vi "SQL_SearchSpareParts.vi"() -> (1 "`Location.Text":string, 2 "Description.Text":string, 3 "ToolCribPN.Text":string)   [LabVIEW 2017]
panel:
  out "ResultQueryString":string
  in  "stop":bool
  in  "Selector":u16(ring)=1 items=["Model", "Make", "ToolCribPN", "Description"]
  in  "Location":u16(ring) items=["12-A-10", "11-B-02", "16-A-03", "15-A-09", "ZARA-A-04", "13-C-02", "11-D-04", "ZARA-A-02", "11-A-02", "RACK-D-06", "11-B-02", "16-A-03", "ZARA-C-08", "ZARA-B-11", "ZARA-B-11", "11-D-09", "15-A-09", "15-A-09", "11-C-04", "ZARA-C-02", "18-C-02", "18-C-02", "18-C-02", "18-C-03", "18-C-03", "18-C-03", "18-C-02", "18-C-05", "ZARA-C-05", "ZARA-C-04", "18-C-03", "18-C-03", "18-C-03", "18-C-03", "18-C-03", "18-C-07", "18-C-07", "15-A-03", "15-C-08", "ZARA-C-09", "ZARA-B-02", "ZARA-B-03", "18-C-14", "RACK-30B-6", "18-C-12", "18-C-14", "18-C-13", "ZARA-B-02", "CARRO-J-02", "ZARA-C-04", "15-C-07", "18-C-14", "18-C-07", "18-C-07", "RACK-30A-1", "11-B-05", "GAV,PAPELE", "16-A-04", "11-B-05", "11-B-06", "11-B-06", "RACK30F-08", "ZARA-A-10", "15-C-11", "15-C-05", "15-B-08", "RACK30C-07", "18-C-07", "15-C-11", "11-C-07", "16-A-12", "16-A-05", "16-A-01", "RACK-7-04", "16-A-09", "15-B-6", "CARRO-B-06", "11-B-03", "ZARA-B-10", "11-B-03", "15-A-16", "15-B-03", "11-B-02", "16-A-01", "15-B-11", "16-A-09", "15-B-11", "15-B-11", "15-B-11", "15-B-12", "15-B-12", "15-A-17", "RACK-30G-4", "11-C-05", "15-B-11", "15-B-11", "RACK-30A-7", "15-B-12", "16-A-04", "RACK-30G-4", "18-C-03", "15-B-03", "11-C-05", "19-D-05", "18-C-07", "16-A-07", "19-A-05", "18-M-05", "19-A-01", "19-A-01", "19-A-01", "19-A-01", "19-A-01", "19-A-01", "19-A-01", "16-A-01", "15-A-01", "19-A-08", "19-A-01", "19-A-01", "19-A-01", "19-A-01", "19-A-01", "19-A-01", "19-A-01", "19-A-01", "19-A-01", "18-C-14", "19-A-02", "19-A-07", "11-D-03", "15-C-03", "18-C-13", "19-A-07", "18-C-14", "19-A-03", "19-A-02", "15-A-01", "16-A-01", "19-D-01", "19-A-02", "19-A-02", "19-A-02", "19-A-03", "19-A-02", "19-A-02", "15-B-10", "15-B-10", "15-B-10", "19-D-07", "19-D-07", "11-D-01", "19-C-01", "19-C-01", "19-C-01", "19-C-01", "19-C-01", "19-C-01", "19-D-03", "19-D-03", "19-D-03", "19-D-03", "19-D-03", "19-D-03", "19-D-03", "16-A-01", "19-D-03", "19-D-03", "19-D-03", "19-D-03", "19-D-03", "19-D-03", "19-D-03", "19-D-03", "19-D-03", "19-D-03", "19-D-03", "19-D-03", "19-D-03", "19-D-03", "19-D-03", "19-D-03", "19-D-08", "19-D-02", "19-D-06", "19-D-05", "19-D-06", "ZARA-L-18", "19-A-03", "19-A-03", "19-D-03", "19-D-03", "19-A-03", "19-A-03", "15-B-08", "19-A-11", "19-A-03", "19-A-03", "19-A-03", "19-A-03", "19-A-06", "RACK-5E-02", "19-B-04", "19-B-07", "PENT.", "18-C-05", "PENT.", "19-A-03", "19-A-03", "15-B-07", "18-M-02", "19-A-03", "19-A-03", "19-A-03", "19-D-10", "19-A-02", "19-A-05", "19-A-05", "19-D-09", "19-A-07", "15-A-04", "15-A-04", "19-D-04", "RACK33B-03", "ZARA-K-12", "15-C-01", "ZARA-K-17", "15-C-01", "15-C-01", "19-A-03", "19-A-04", "19-A-04", "15-B-11", "19-A-04", "19-A-04", "19-A-04", "19-A-10", "19-A-04", "19-D-02", "CARRO-B-03", "15-B-05", "11-C-01", "ZARA-K-08", "ZARA-K-08", "ZARA-K-08", "11-C-01", "ZARA-K-08", "11-C-01", "ZARA-K-12", "11-C-01", "15-C-01", "ZARA-K-18", "ZARA-K-16", "ZARA-K-08", "19-A-05", "11-C-01", "15-B-04", "19-C-02", "15-C-05", "17-D-11", "GAV QUIM 1", "15-B-10", "17-D-08", "17-D-11", "15-C-04", "15-B-01", "15-B-04", "11-G-01", "11-G-01", "11-G-01", "18-C-14", "ZARA-S-03", "15-C-02", "17-D-01", "15-A-02", "19-A-04", "19-A-04", "18-C-05", "19-A-04", "18-C-05", "18-C-05", "18-M-03", "RACK-4D-01", "RACK30G-03", "19-A-04", "19-A-04", "19-A-04", "CARRO-H-03", "RACK-11K-8", "CARRO-B-01", "15-B-06", "19-A-11", "19-A-09", "18-M-01", "19-A-11", "15-B-11", "ZARA-K-22", "CARRO-H-02", "ZARA-L-05", "RACK33B-02", "RACK33B-02", "RACK33B-02", "CARRO-A-06", "CARRO-A-06", "CARTO-QUIM", "ZARA-K-09", "ZARA-L-05", "ZARA-L-05", "ZARA-L-05", "CARRO-A-03", "19-A-02", "CARRO-A-06", "CARRO-A-06", "CARRO-A-06", "ZARA-V-02", "ZARA-V-02", "ZARA-K-20", "ZARA-E-02", "CARRO-L-03", "ZARA-K-16", "ZARA-K-07", "19-C-06", "CARRO-A-06", "19-C-06", "CARRO-A-06", "CARRO-A-06", "ZARA-K-21", "ZARA-K-20", "19-B-04", "CARRO-H-03", "RACK-33A-1", "ZARA-K-16", "ZARA-K-16", "19-C-04", "19-C-04", "CARRO-H-02", "ZARA-L-05", "18-M-01", "11-B-08", "16-A-02", "CARRO-H-04", "ZARA-T-01", "ZARA-S-05", "ZARA-S-05", "ZARA-U-03", "ZARA-K-06", "ZARA-K-05", "13-C-02", "ZARA-L-16", "ZARA-D-01", "18-M-02", "CARRO-B-05", "15-A-07", "11-C-07", "CARRO-A-12", "15-C-02", "ZARA-L-17", "CARRO-B-12", "ZARA-T-02", "ZARA-L-05", "ZARA-Q-03", "ZARA-F-02", "ZARA-F-02", "ZARA-K-20", "11-D-01", "ZARA-K-14", "11-D-02", "ZARA-K-13", "ZARA-K-06", "ZARA-L-17", "ZARA-K-06", "ZARA-K-06", "ZARA-K-13", "ZARA-K-06", "ZARA-K-16", "ZARA-K-16", "ZARA-K-18", "ZARA-K-05", "ZARA-D-02", "ZARA-K-05", "ZARA-K-05", "CARRO-A-05", "ZARA-K-05", "ZARA-K-05", "11-B-03", "ZARA-K-18", "ZARA-L-02", "CARRO-I-01", "ZARA-L-16", "ZARA-L-02", "ZARA-K-13", "11-D-02", "15-B-04", "13-C-03", "ZARA-V-02", "ZARA-U-09", "17-D-02", "CARRO-H-04", "ZARA-L-01", "ZARA-K-08", "15-B-10", "ZARA-D-03", "ZARA-L-01", "ZARA-K-12", "15-A-04", "15-B-07", "ZARA-D-02", "11-G-01", "CARRO-G-03", "11-D-02", "CARRO-G-03", "ZARA-K-06", "ZARA-J-02", "ZARA-K-06", "ZARA-K-11", "ZARA-S-03", "11-D-02", "ZARA-K-13", "ZARA-U-06", "ZARA-K-13", "ZARA-K-13", "15-B-06", "ZARA-L-13", "11-B-02", "11-B-02", "11-C-07", "11-C-07", "11-D-01", "11-C-07", "11-D-01", "11-D-01", "ZARA-L-04", "ZARA-K-10", "ZARA-L-13", "11-C-01", "11-D-02", "ZARA-L-04", "ZARA-L-07", "ZARA-K-14", "11-D-01", "15-B-05", "ZARA-K-10", "ZARA-M-04", "15-C-02", "ZARA-K-14", "ZARA-M-04", "ZARA-M-04", "ZARA-M-04", "ZARA-M-04", "ZARA-M-04", "ZARA-K-21", "15-C-02", "ZARA-D-06", "ZARA-L-06", "ZARA-L-06", "ZARA-L-06", "15-B-06", "15-B-05", "15-B-05", "CARRO-G-05", "18-C-06", "ZARA-J-05", "19-D-01", "ZARA-Q-04", "18-C-09", "CARRO-A-01", "11-C-01", "CARRO-J-02", "CARRO-H-03", "CARRO-L-03", "CARRO-H-03", "CARRO-L-03", "ZARA-P-06", "ZARA-K-10", "ZARA-L-08", "CARRO-E-02", "ZARA-L-03", "ZARA-Q-04", "11-C-01", "ZARA-M-08", "CARRO-G-10", "CARRO-G-10", "CARRO-G-10", "CARRO-G-10", "11-A-06", "ZARA-S-03", "ZARA-U-09", "ZARA-L-13", "ZARA-L-10", "ZARA-K-06", "CARRO-B-02", "CARRO-H-03", "ZARA-L-01", "ZARA-K-14", "CARRO-G-10", "ZARA-M-08", "PENT.", "ZARA-F05-1", "17-D-01", "14-B-06", "ZARA-K-22", "ZARA-L-15", "G.QUIMICOS", "18-M-04", "RACK30F-06", "15-C-06", "15-A-17", "11-G-04", "ZARA-K-17", "ZARA-K-11", "18-M-01", "RACK30C-04", "11-B-06", "17-D-06", "RACK30F-06", "GAV1,QUIMI", "18-M-03", "15-C-11", "11-B-04", "15-A-02", "15-A-04", "RACK-3C-02", "ZARA-L-15", "RACK-4D-07", "17-D-05", "15-C-04", "15-A-01", "RACK-D4-07", "18-C-10", "CARRO-B-10", "CARRO-B-10", "CARRO-B-10", "CARRO-B-10", "ZARA-L-05", "CARRO-B-10", "RACK-D4-03", "ZARA-L-10", "11-C-03", "18-M-04", "18-C-10", "15-C-04", "CARRO-G-01", "17-D-11", "11-C-01", "11-C-03", "15-C-10", "15-A-01", "ZARA-K-16", "14-B-05", "17-D-06", "ZARA-L-16", "11-B-04", "17-D-10", "15-B-10", "ZARA-C-01", "RACK-5E-01", "15-A-14", "ZARA-L-10", "ZARA-L-10", "ZARA-L-10", "ZARA-Q-04", "15-C-03", "15-C-03", "11-C-06", "ZARA-L-15", "13-C-05", "ZARA-L-14", "ZARA-M-05", "ZARA-F-16", "17-D-02", "15-A-08", "17-D-01", "17-D-01", "ZARA-L-10", "17-D-01", "RACK-B-00", "RACK-B-00", "RACK-B-00", "11-C-01", "CARRO-A-04", "17-D-06", "15-B-08", "15-B-08", "15-B-08", "15-B-08", "19-D-04", "19-D-04", "17-D-08", "13-C-01", "13-C-01", "ZARA-L-07", "15-B-03", "11-B-04", "18-C-06", "17-D-01", "ZARA-L-15", "ZARA-L-15", "11-B-04", "15-A-11", "ZARA-M-08", "ZARA-K-15", "14-B-09", "17-D-02", "18-M-03", "15-B-02", "15-B-02", "15-B-02", "ZARA-M-06", "ZARA-S-04", "17-D-02", "ZARA-L-19", "GAV-QUIM1", "15-C-06", "18-C-06", "CARRO-C-02", "CARRO-C-02", "ZARA-J-01", "11-B-08", "ZARA-M-03", "ZARA-F-17", "ZARA-M-03", "ZARA-M-03", "ZARA-J-01", "ZARA-E-04", "ZARA-M-10", "ZARA-M-08", "ZARA-M-08", "15-B-02", "15-B-02", "15-B-02", "ZARA-J-01", "12-A-10", "15-B-11", "15-C-05", "11-A-02", "14-B-09", "CARRO-G-06", "CARRO-G-06", "15-C-07", "14-B-09", "11-A-02", "CARRO-G-06", "11-A-02", "CARRO-G-06", "ZARA-J-01", "ZARA-M-10", "CARRO-A-04", "CARRO-G-06", "CARRO-A-04", "ZARA-P-04", "CARRO-G-06", "11-D-04", "11-D-04", "11-D-04", "CARRO-A-04", "CARRO-A-04", "CARRO-G-06", "11-B-07", "PENDIENTE", "PENDIENTE", "CARRO-C-04", "ZARA-M-10", "14-B-05", "CARRO-A-02", "CARRO-A-02", "14-B-09", "CARRO-B-12", "CARRO-J-02", "15-C-06", "15-C-04", "ZARA-K-07", "CUARTO NUV", "ZARA-P-05", "ZARA-N-13", "ZARA-N-03", "ZARA-N-04", "ZARA-N-02", "ZARA-O-11", "ZARA-M-10", "CARRO-A-01", "15-B-02", "11-C-02", "ZARA-N-01", "ZARA-N-01", "ZARA-N-01", "ZARA-N-01", "ZARA-N-01", "15-A-16", "11-D-02", "RACK-D-5", "ZARA-N-12", "ZARA-N-12", "18-C-08", "18-C-08", "CARRO-B-03", "12-A-05", "15-C-04", "15-C-04", "11-D-10", "ZARA-N-01", "18-M-07", "ZARA-N-13", "ZARA-N-13", "ZARA-T-06", "ZARA-T-06", "ZARA-T-06", "ZARA-T-06", "ZARA-T-06", "ZARA-T-06", "ZARA-O-14", "CARRO-A-03", "CARRO-A-03", "CARRO-A-03", "CARRO-A-03", "CARRO-A-03", "CARRO-A-03", "CARRO-A-03", "CARRO-A-03", "CARRO-A-03", "CARRO-A-03", "CARRO-A-03", "CARRO-A-03", "CARRO-A-03", "ZARA-N-04", "ZARA-N-04", "CARRO-A-03", "CARRO-A-03", "CARRO-A-03", "11-C-01", "11-C-02", "11-C-02", "ZARA-N-12", "ZARA-N-04", "ZARA-N-04", "ZARA-N-04", "ZARA-N-12", "11-C-01", "CARRO-A-03", "ZARA-T-06", "ZARA-T-06", "ZARA-T-06", "ZARA-T-06", "ZARA-T-06", "CARRO-A-03", "11-D-01", "11-D-01", "11-C-06", "11-D-01", "CARRO-A-03", "CARRO-B-05", "15-C-03", "11-D-02", "ZARA-P-04", "ZARA-O-09", "ZARA-N-13", "ZARA-N-13", "ZARA-N-13", "ZARA-P-02", "ZARA-N-15", "ZARA-U-01", "11-B-05", "CARRO-A-04", "ZARA-P-04", "ZARA-O-13", "ZARA-O-13", "ZARA-O-14", "ZARA-O-13", "ZARA-O-13", "ZARA-O-13", "ZARA-O-13", "11-C-01", "ZARA-T-07", "ZARA-T-07", "ZARA-T-07", "ZARA-T-07", "ZARA-T-07", "ZARA-T-07", "CARRO-L-02", "CARRO-L-02", "ZARA-T-03", "ZARA-P-04", "ZARA-O-13", "CARRO-B-12", "17-D-07", "ZARA-T-07", "ZARA-T-07", "CARRO-K-06", "CARRO-K-09", "ZARA-T-03", "ZARA-T-03", "ZARA-T-06", "ZARA-T-04", "ZARA-T-04", "ZARA-T-04", "ZARA-T-04", "ZARA-T-04", "ZARA-T-04", "CARRO-B-12", "CARRO-B-12", "CARRO-B-12", "CARRO-B-12", "ZARA-T-04", "ZARA-T-04", "ZARA-T-04", "ZARA-T-05", "ZARA-T-05", "ZARA-T-05", "ZARA-T-05", "ZARA-T-05", "ZARA-T-07", "ZARA-T-07", "ZARA-T-07", "ZARA-T-07", "ZARA-T-07", "ZARA-T-07", "ZARA-T-07", "15-A-16", "13-C-03", "CARRO-B-04", "CARRO-A-02", "CARRO-A-02", "11-D-03", "ZARA-U-01", "ZARA-T-09", "CARRO-H-03", "17-D-02", "ZARA-U-04", "ZARA-U-04", "ZARA-U-04", "ZARA-U-04", "ZARA-U-04", "ZARA-U-04", "CARRO-K-02", "CARRO-K-02", "ZARA-U-04", "CARRO-K-09", "ZARA-U-04", "ZARA-U-04", "ZARA-T-02", "18-C-17", "CARRO-K-09", "11-D-03", "RACK30B-07", "11-B-03", "CARRO-K-09", "CARRO-B-11", "CARRO-B-11", "CARRO-B-11", "CARRO-B-11", "CARRO-B-11", "CARRO-G-09", "CARRO-G-09", "CARRO-G-09", "CARRO-G-09", "CARRO-C-05", "15-B-06", "CARRO-G-08", "15-A-04", "CARRO-G-12", "CARRO-B-07", "11-D-07", "14-B-02", "11-D-04", "PEND.", "15-B-08", "15-B-08", "CARRO-G-11", "11-D-02", "CARRO-G-01", "11-D-02", "CARRO-G-11", "CARRO-G-11", "CARRO-G-12", "CARRO-G-12", "PEND.", "PEND.", "15-B-07", "CARRO-G-12", "CARRO-K-05", "CARRO-K-05", "RACK33B-02", "15-B-06", "CARRO-A-10", "CARRO-A-10", "CARRO-A-11", "CARRO-A-11", "CARRO-A-11", "CARRO-A-11", "CARRO-G-07", "CARRO-G-07", "CARRO-G-07", "CARRO-G-07", "CARRO-G-07", "CARRO-G-07", "CARRO-G-07", "18-C-03", "RACK-I-04", "CARRO-B-07", "CARRO-B-07", "CARRO-A-12", "CARRO-A-12", "CARRO-A-12", "11-D-07", "15-B-08", "11-D-03", "18-M-08", "11-D-07", "18-M-09", "15-B-08", "CARRO-B-10", "CARRO-G-11", "CARRO-G-11", "CARRO-B-04", "CARRO-G-06", "CARRO-G-11", "CARRO-G-06", "ZARA-O-04", "EN CUARTO", "CARRO-D-03", "CARRO-G-11", "15-B-02", "ZARA-O-04", "19-C-02", "ZARA-P-07", "ZARA-O-04", "CARRO-B-10", "18-C-10", "CARRO-K-05", "CARRO-K-05", "CARRO-K-05", "CARRO-K-05", "CARRO-K-05", "CARRO-K-05", "CARRO-K-05", "CARRO-K-05", "CARRO-K-05", "15-C-04", "ZARA-Q-09", "PENDIENTE", "CARRO-B-06", "CARRO-B-06", "CARRO-K-03", "CARRO-K-05", "CARRO-K-05", "CARRO-K-05", "CARRO-K-05", "CARRO-K-05", "CARRO-K-05", "CARRO-K-05", "CARRO-A-08", "PEND.", "CARRO-B-09", "CARRO-K-07", "ZARA-Q-09", "CARRO-K-03", "CARRO-K-03", "15-C-04", "15-B-03", "11-B-05", "CARRO-K-05", "CARRO-K-06", "PEND.", "PEND.", "15-B-09", "CARRO-A-07", "CARRO-A-07", "CARRO-A-07", "CARRO-A-07", "CARRO-A-07", "CARRO-A-07", "CARRO-A-07", "CARRO-A-07", "ZARA-W-04", "PEND.", "ZT-***", "CARRO-K-09", "CARRO-K-09", "ZARA-E-01", "ZARA-E-01", "ZARA-E-03", "ZARA-E-01", "ZARA-E-01", "ZARA-E-03", "ZARA-E-03", "", "CARRO-B-12", "18-M-04", "15-B-01", "PEND.", "ZARA-O-06", "ZARA-O-06", "ZARA-O-06", "ZARA-O-06", "ZARA-O-06", "ZARA-O-06", "ZARA-O-06", "ZARA-O-06", "ZARA-O-06", "ZARA-O-06", "ZARA-O-06", "ZARA-O-06", "ZARA-O-06", "ZARA-O-06", "ZARA-O-06", "ZARA-O-06", "ZARA-O-06", "ZARA-O-06", "ZARA-O-06", "ZARA-O-06", "ZARA-O-07", "ZARA-O-07", "ZARA-O-07", "ZARA-O-07", "ZARA-O-07", "ZARA-O-07", "ZARA-O-07", "ZARA-O-07", "ZARA-O-07", "ZARA-O-07", "ZARA-O-07", "ZARA-O-07", "ZARA-O-06", "ZARA-O-06", "ZARA-O-06", "ZT-*****", "ZT-R2-02-C", "ZT-*****", "ZT-R2-03-A", "ZT-G7-01", "ZT-G6-01", "ZARA-T-08", "ZARA-U-07", "ZT-****", "ZT-PISO-2", "ZT-R2-05-B", "ZT-PISO-1", "ZT-****", "ZT-*****", "ZT-*****", "ZT-R5-04-B", "ZT-*****", "ZARA-T-08", "ZARA-T-08", "ZARA-T-08", "CARRO-G-05", "CARRO-G-10", "CARRO-G-10", "CARRO-G-10", "CARRO-G-10", "CARRO-G-10", "CARRO-G-10", "CARRO-G-10", "CARRO-G-10", "CARRO-G-10", "CARRO-G-10", "CARRO-G-10", "CARRO-G-10", "CARRO-G-10", "CARRO-G-10", "CARRO-G-10", "CARRO-G-10", "CARRO-G-10", "CARRO-G-10", "CARRO-G-10", "ZARA-U-07", "ZARA-U-07", "ZARA-U-07", "ZARA-U-07", "ZARA-U-07", "ZARA-U-07", "ZARA-U-07", "ZARA-U-07", "ZARA-U-07", "ZARA-U-07", "ZARA-U-07", "ZARA-U-07", "ZARA-U-07", "ZARA-U-07", "ZARA-U-07", "ZARA-U-07", "ZARA-U-07", "ZARA-U-07", "CARRO-G-10", "CARRO-G-10", "CARRO-G-10", "PENDIENTE", "PENDIENTE", "PENDIENTE", "PENDIENTE", "PENDIENTE", "PENDIENTE", "PENDIENTE", "PENDIENTE", "ZARA-Q-07", "PENDIENTE", "CARRO-G-10", "CARRO-G-10", "CARRO-G-10", "11-D-03", "ZARA-R-03", "CARRO-K-07", "ZARA-U-08", "ZARA-Q-07", "ZARA-W-03", "ZT-******", "ZT-*****", "ZT-*****", "ZT-*****", "ZT-G3-E", "CARRO-G-05", "CARRO-G-05", "CARRO-G-05", "CARRO-G-05", "CARRO-G-05", "CARRO-G-05", "ZT-******", "ZT-******", "ZT-G5-C", "ZT-******", "ZT-******", "18-M-06", "ZT-*****", "ZT-*****", "ZT-******", "ZT-******", "ZT-******", "ZT-******", "ZT-******", "ZT-G5-B", "15-C-07", "ZT-*****", "ZT-*****", "ZT-******", "ZT-******", "ZT-R3-01-A", "ZT-R1-05-A", "ZT-R6-03-C", "ZT-R1-04-B", "ZT-G5-B", "ZT-R1-04-A", "ZT-******", "ZT-G5-C", "ZT-G5-C", "ZT-G0-B", "ZT-G0-B", "ZT-G0-B", "CARRO-K-02", "CARRO-B-12", "CARRO-B-12", "CARRO-K-07", "CARRO-K-07", "CARRO-K-01", "CARRO-K-01", "CARRO-K-01", "CARRO-K-01", "CARRO-K-01", "CARRO-K-01", "CARRO-K-01", "CARRO-K-01", "CARRO-K-01", "CARRO-K-01", "CARRO-K-01", "CARRO-K-01", "CARRO-K-01", "CARRO-K-01", "CARRO-K-01", "CARRO-K-01", "CARRO-K-01", "CARRO-K-01", "CARRO-K-01", "CARRO-K-01", "CARRO-K-01", "CARRO-K-01", "CARRO-K-01", "CARRO-K-01", "CARRO-K-01", "CARRO-K-01", "CARRO-K-01", "CARRO-K-01", "CARRO-K-01", "CARRO-A-05", "CARRO-A-05", "CARRO-A-05", "CARRO-A-05", "CARRO-A-05", "CARRO-A-05", "ZT-*****", "ZT-*****", "ZARA-Q-07", "ZARA-Q-07", "ZARA-Q-07", "ZARA-Q-07", "ZARA-Q-07", "ZARA-Q-07", "ZARA-Q-07", "ZARA-Q-07", "CARRO-A-01", "CARRO-K-01", "CARRO-A-05", "CARRO-K-02", "ZARA-Q-11", "PEND.", "ZARA-Q-11", "PEND.", "PEND.", "PEND.", "PEND.", "PEND.", "11-D-06", "PENDIENTE", "ZARA-U-08", "ZARA-U-08", "ZARA-U-08", "ZARA-U-08", "ZARA-U-08", "ZARA-U-08", "ZARA-U-08", "ZARA-U-08", "ZARA-U-08", "ZARA-U-08", "ZARA-U-08", "PEND.", "ZARA-Q-08", "ZARA-R-03", "ZARA-R-03", "ZARA-R-04", "ZARA-R-04", "ZARA-R-04", "FACILITIES", "FACILITIES", "FACILITIES", "PENDIENTE.", "PENDIENTE.", "RACK", "RACK", "15-C-07", "G.QUIM", "17-D-02", "15-B-02", "14-B-11", "14-B-03", "PEND.", "15-B-04", "18-M-09", "ZARA-A-08", "15-B-09", "MP01", "15-A-11", "11-B-01", "11-B-01", "11-C-03", "11-C-08", "11-D-08", "13-C-03", "ZARA-B-08", "15-B-06", "18-M-09", "18-M-09", "15-B-07", "14-B-01", "ZARA-B-14", "11-C-03", "15-B-06", "11-D-08", "15-B-11", "ZARA-C-02", "RACK-E5-05", "15-C-07", "ZARA-A-10", "15-B-11", "ZARA-C-03", "18-M-05", "11-G-06", "15-B-10", "30-A-03", "11-G-06", "15-C-03", "15-A-06", "RACK-33B-1", "11-G-05", "14-B-01", "15-C-07", "RACK-33A-2", "RACK-3C-8", "11-A-01", "11-A-01", "11-A-01", "15-C-10", "15-C-10", "11-A-02", "ZARA-B-09", "ZARA-B-03", "18-C-09", "ZARA-A-08", "ZARA-C-08", "11-A-02", "GAVETA-A-2", "ZARA-B-08", "GAVETA-A-2", "GAV,PAPELE", "17-D-07", "ZARA-B-09", "11-A-03", "18-C-09", "18-C-09", "11-A-02", "GAV-QUI-2", "11-A-05", "ZARA-B-09", "11-A-03", "11-A-03", "CARRO-J-02", "11-A-03", "MANT-6", "RACK MTLS", "18-M-05", "11-A-07", "11-A-02", "11-A-06", "14-B-01", "ZARA-B-08", "11-A-07", "11-A-07", "11-A-07", "11-A-06", "11-B-07", "11-B-07", "RACK-G7-01", "", "11-A-07", "11-A-07", "PAP-03", "16-A-01", "16-A-01", "ZARA-C-04", "16-A-09", "RACK-H8-01", "16-A-02", "16-A-02", "11-A-06", "ZARA-A-05", "ZARA-B-08", "ZARA-K-17", "ZARA-E-02", "RACK-30C-2", "ZARA-B-13", "11-G-01", "11-G-01", "", "11-G-01", "ZARA-B-13", "ZARA-B-11", "11-B-07", "11-G-01", "11-G-01", "GAV-B-05", "RACK33A-02", "ZARA-C-04", "16-A-09", "ZARA-B-10", "16-A-02", "16-A-11", "GAV.QUIMIC", "14-B-01", "18-C-08", "18-C-08", "GAV-A-2", "MANT-8", "CARRO-I-03", "ZARA-C-12", "ZARA-C-12", "ZARA-C-11", "GAB-B-02", "16-A-02", "16-A-12", "18-C-09", "13-C-05", "15-C-07", "19-C-07", "11-G-02", "ZARA-B-13", "ZARA-B-13", "11-G-03", "11-G-03", "11-G-03", "11-G-03", "13-C-07", "ZARA-B-09", "11-B-03", "15-A-16", "15-A-16", "GAV-B-05", "ZARA-B-11", "15-B-06", "GAV-B-03", "GAV-B-03", "GAV-B-03", "GAV-B-07", "11-G-02", "11-B-03", "ZARA-A-03", "11-B-03", "ZARA-A-03", "ZARA-A-03", "ZARA-A-05", "11-B-09", "11-B-02", "GAV-B-03", "GAV-B-07", "15-C-02", "ZARA-B-11", "15-A-04", "ZARA-C-02", "15-C-4", "ZARA-C-02", "ZARA-C-02", "11-B-03", "11-G-04", "11-B-09", "ZARA-A-05", "11-B-09", "11-B-09", "ZARA-A-05", "ZARA-A-08", "11-C-02", "11-D-05", "12-A-06", "11-B-02", "11-B-02", "18-M-07", "ZARA-A-05", "11-C-06", "ZARA-A-05", "GAV-B-10", "GAV-B-07", "GAV-B-09", "GAV-B-03", "ZARA-B-09", "GAV-B-09", "GAV-B-09", "11-D-05", "15-C-08", "GAV-QUIM", "GAV-QUIM", "ZARA-B-11", "11-C-06", "16-A-03", "ZARA-A-04", "11-B-02", "11-B-02", "ZARA-L-01", "ZARA-T-09", "14-B-11", "ZARA-B-11", "11-C-06", "12-A-05", "RACK-4D-09", "15-C-01", "ZARA-C-01", "15-B-10", "15-B-10", "ZARA-B-15", "11-B-04", "ZARA-C-07", "15-C-04", "RACK-11K-2", "ZARA-B-13", "17-D-04", "15-A-04", "17-D-07", "18-C-10", "11-D-02", "11-A-03", "CARRO-D-02", "CARRO-G-11", "18-C-05", "ZARA-E-05", "11-C-01", "ZARA-V-05", "CARRO-B-05", "ZARA-R-02", "ZARA-F-17", "17-D-07", "ZT-****", "ZARA-N-09", "15-A-16", "15-A-16", "19-A-01", "11-B-04", "CARRO-C-02", "ZARA-X-03", "19-A-01", "16-A-09", "ZARA-N-13", "15-B-04", "13-C-05", "19-A-08", "11-G-01", "CARRO-K-05", "19-A-02", "11-C-02", "CARRO-G-06", "15-C-08", "CARRO-A-03", "18-C-10", "ZARA-K-14", "ZARA-T-07", "ZARA-T-07", "ZARA-T-08", "ZARA-K-08", "PENDIENTE", "ZARA-R-06", "ZARA-R-06", "ZARA-R-06", "ZARA-R-06", "ZARA-R-06", "ZARA-R-06", "ZARA-R-06", "ZARA-R-06", "ZARA-R-06", "ZARA-R-06", "ZARA-R-06", "ZARA-R-06", "ZARA-R-06", "ZARA-R-06", "ZARA-R-06", "ZARA-R-06", "ZARA-R-06", "ZARA-R-06", "ZARA-R-06", "ZARA-E-06", "ZARA-X-08", "ZARA-R-08", "ZARA-R-08", "ZARA-R-08", "ZARA-E-05", "ZARA-E-05", "ZARA-E-05", "ZARA-E-05", "ZARA-E-07", "ZT-****", "ZT-****", "ZARA-R-07", "11-B-05", "ZT-****", "ZT-****", "ZT-****", "ZT-****", "ZT-****", "ZT-****", "ZT-****", "ZT-****", "ZT-****", "ZT-****", "ZT-****", "ZT-****", "ZARA-N-09", "ZARA-X-03", "ZARA-X-03", "ZARA-X-03", "ZARA-X-03", "ZARA-X-04", "ZARA-X-07", "ZARA-X-07", "ZARA-X-01", "ZARA-X-03", "ZARA-A-12", "ZARA-X-06", "11-A-03", "ZARA-Y-04", "11-A-03", "ZARA-X-01", "ZARA-O-11", "ZARA-Q-03", "CARRO-A-02", "ZARA-R-4", "ZARA-A-07", "15-B-10", "15-B-10", "ZARA-X-06", "15-C-01", "ZARA-N-05", "ZARA-N-05", "ZARA-N-05", "ZARA-N-05", "ZARA-N-05", "ZARA-X-07", "ZARA-N-05", "ZARA-N-09", "CARRO-A-02", "ZARA-B-15", "ZARA-N-05", "GAV-QUIM", "ZARA-N-05", "ZARA-E-04", "14-B-05", "15-A-12", "ZARA-Q-07", "ZARA-Q-07", "ZARA-E-06", "PENDIENTE.", "ZARA-X-09", "ZARA-N-09", "ZARA-T-03", "14-B-03", "14-B-03", "GAV-QUIM-2", "ZARA-Y-04", "PENDIENTE", "CARRO-B-01", "ZARA-M-09", "ZARA-M-09", "PEND.", "CARRO-B-01", "ZARA-J-11", "ZARA-J-11", "ZARA-J-11", "CARRO-B-01", "CARRO-B-01", "CARRO-B-01", "CARRO-B-01", "CARRO-B-01", "CARRO-B-01", "PEND.", "PEND.", "PEND.", "PEND.", "PEND.", "PEND.", "ZARA-C-02", "CARRO-G-05", "ZARA-X-09", "11-B-05", "15-A-16", "15-A-16", "15-A-16", "11-B-04", "ZARA-B-13", "15-B-04", "ZARA-B-13", "15-B-08", "11-D-08", "15-B-05", "ZARA-C-01", "ZARA-C-01", "ZARA-C-01", "ZARA-C-01", "ZARA-C-01", "ZARA-C-01", "15-B-12", "ZARA-C-01", "15-C-04", "14-B-05", "15-B-05", "15-C-01", "ZARA-C-07", "18-M-04", "ZARA-C-07", "CARRO-G-05", "ZARA-N-09", "CARRO-B-12", "", "ZARA-K-08", "ZARA-T-07", "PEND.", "CARRO-B-01", "CUARTO NUV", "PEND.", "RACK-E5-03", "11-D-03"]
  in  "Description":u16(ring) items=["TARJETA USB-6525,8  #779640-01", "GKS-005 206  396 A 2000 TEST PROBE", "BUMBER MISUMI UTTM-D19-A6-L12-C10-V2-VL5", "BALLUF MAGNETIC  BMF 307K-PS-C-2-SA2-S49", "RELAY SOCKET FINDER 97.01 -250V,16A", "MOUSE DELL 09RRC7", "BALERO 6900Z NTN", "BALERO 696Z EZO", "G62946-1 RETAINING CAP, JOURNAL SLIDE", "FORMATO QRAP (60 X 90 A DOS TINTAS)", "LBC-2K   2000 LBS (S/N 332979 ) CELDA", "JOINT SHAFT 229J014161B  SCM 435", "FILTER ELEMENT #09913740", "USB-DI096/50 DIGITAL I/O MODULE", "05-092 SURGE BOARD WITH REMOVEABLE RELAY", "01-DT9814 A/D ASSY", "SENSOR INDUCTIVO  IFM IE5091", "SENSOR INDUCTIVO  IFM IE5090", "SENSE CABLE  IPB5000A   4-37229-01", "TNPGB0309CN1 -TINA 06 PIN GUIDE BUSH  NS", "TNEPBD060950- TINA EP 06 BODY (ONLY)NS", "FABRICACION DE INSERTO DERECHO 069 A", "FABRICACION DE INSERTO IZQUIERDO 069 C", "5937K79 LEVER-HANDLE BLOWGUN WITH 3\"", "7013A19 T6 TORX BIT, 1/4\" HEX SHANK", "7-2836329-7 SPARE PARTS KIT", "ORING 2.5 X 90", "1409B  BRASS BRUSH 3/8", "EP-SWR37--90 YELLOW SPRING 37X26X90 MM", "EP -93-1225 RED SPRING 12X6X25 MM", "ANVIL, COMBINATION  7-1633927-8", "CRIMPER, INSULATION F PREMIUM 4-2119784-", "CRIMPER, WIRE PREMIUM  2-1490019-0", "1825-0099 RESORTE DE TENSION", "1825-0098 RESORTE DE TENSION", "45-045-0109 CONTACT PIN,.32 HARD SPRING", "2119791-5 DEPRESSOR, WIRE", "IZ5048 EFECTOR 3MM PNP-IZ9301-BPKG/2M", "079340-98013 LOCTITE 98013 CA DIAPHRAGM", "G7918671 COLLECTOR BAG, 2.5 CU. FT.", "PHD RAS125X90-DB-M-PB-Q10ROTARY ACTUADOR", "CDQSB25-90DCM  CILINDRO COMPACTO 250X90", "WIRE FIT PLATE 4B297732P0101-0", "P/N 36110975 200 UF 2000 VDC OIL CAP.", "100422701 9353 12-BIT CHARGE CONTROL 230", "BALERO F695ZZ", "CONECTOR BNC PERMASEAL PARA RG59", "779675-01  USB -6210 DISPOSITIVO DE E/S", "DAW-42309 CDA1B50-100-A54L- AIR CYLINDER", "8938A44 THREE-SIDED FLAT BELLOW 8-1/8\"X2", "CR5395-EH-ACV-110-X-CD-ELR-I DC CURRECT", "TIMING BELT B100S3M279(K)", "Y5 90029 TIP,1/2, UNIVERS L, UNDER UT", "Y5 90002 NVIL, 1/2", "SWITCH 16 PUERTOS TP-RJ45 2832849", "TENSION ARMTYPE 6L HK0109", "LLAVEROS STD Y MM EN PUNTA BOLA 20899", "D-Y59BL SENSOR", "CUTTER (A) 4B297720P0101-0", "FELT 4MK20945-0-01E", "CUTTER (B) 4B297721P0101-0", "GUANTE GRIS DE NYLON #SK-GGPU-LG TALLA 9", "C104HS/PCI-DB9M 4 PORT RS-232 BOARD WITH", "CP-104EL-A-DB9M 4-PORT RS-232-LOW PROFIL", "079340-98389 LOCTITE PLYETHLN TPRD, TIP", "410192-0010 CALSET JIG (6TH AXIS)", "589611-86 ENCODERS HEIDENHAIN ERN 120 50", "F93842-C5672 INNER SHIELD SHEAR BLADE", "TEST PROBE 3105-03-B   AZ 10059-000X/18", "RELAY SOCKET 27E892  46F3588", "VALVULA 5/3 A 24 V SY9320-5LZ-C10", "9TRASDULT03011 TRANSDUCER", "ELECTRODE 227H064319B C1720P", "# 140.098 HOTWIND PREMIUM HOT AIR BLOWER", "MGPM12-10ZD-A93VL CILINDRO PLANO CON GUI", "GKS-005 206 396 A 3000 TEST PROBE", "FS-096-BMMTW DBL ACTING SINGLE END ROD 1", "K-B-FS-W-09 KIT DE REPARACION P/CIL. DIA", "ZEBRA-REPLACEMENT PRINTHEAD 105934-038", "BALEROS F695ZZ", "HSS-005 306 396 A 5000 HIGH-CURRENT PROB", "NAVAJA INTELIGENTE (MASTER 101199)", "7396A76 TORX BIT, 1/4\" HEX SHANK  2-3/4\"", "FABRICACION DE PIN #MA190-1", "SPC046-M9 PORTAELECTRODOS INFERIOR", "MSC-4B674499 P0 101 BLADE", "B-J11008-C4509 LEAD GUIDE SLIDE", "B-K93310 NOSE PIECE ASSEMBLY-WIRE CLAMP", "B-L93019 CLAMP ROD", "K94350-45 FLIER ARM", "B-73069 POSITIONER BARREL", "079340-97114 LOCTITE 97114 3/8IN AIR", "4-39621-01 FINAL ASSY, EZ AIR, SINGLE", "K93026-C5672 INNER SHIELD  K93027-C5672", "C-K93223-C5105L LEAD GUIDE RETAINER", "C-K93223-C5105R LEAD GUIDE RETAINER", "CCB-84901-2001-05  COGNEX X-CODED", "RC 01-059-1771-715 PEELE194 TS 06", "0030297 BLADE (G333/ALPHA 4XX)", "3842503590 AC MOTOR,220-420/50", "MSC - 4B781906P0101-0 CUTTER BLADE (B)", "MARTOR REPLACEMENT BLADES MOD. 199", "MECHANICAL ASSEMBLY 2119580-1", "MXQ20L-100B-M9BL MESA DESLIZANTE", "WIRE HOLDER (A) #MSC-3B739838 P0101-0", "#BNR17G08-BMY003-P029 FIXT P/ENSAMBLE", "#G43633 98475 GAUGE MEDICION SPLINE", "#G43633 98476 GAUGE MEDICION SPLINE", "1-1320908-0 SPACER, STRIP GUIDE", "2119805-1 SHEAR HOLDER, FRONT, CUT", "1-2119781-0 DEPRESSOR, SHEAR", "3-2119784-4 CRIMPER, INSULATION", "9-1633305-0 CRIMPER,WIRE PREMIUM.", "2-2119784-5 CRIMPER, INSUL O PREMIUM", "2-1333229-2 ANVIL, COMBINATION SPECIAL", "MSC-3B359797 P0101-0 START WIRE HOOKING", "BES M08MI-PSC20B-SA9G   BES003P", "0024955 CABLE SET, MAIN VALVE (G333)", "2119943-1 WASHER, SPACER", "2119959-2 ASSEMBLY, STRIP GUIDE", "1320928-5 STRIP GUIDE", "2119799-1 HOLDER, FEED FINGER,AF", "318059-9  FLOATING SHEAR, FRONT", "2119799-1 HOLDER, FEED FINGER, AF", "2119806-2 INSERT, SHEAR", "2119805-4 SHEAR HOLDER, FRONT, CUT", "2119781-6 DOPRESSOR, SHEAR.", "COMPRESSON SPRING SPR-4B648792 P0101-0", "0037947 WASHER,SPECIAL,CUTHEAD", "0044549 BELT,TOOTHED,GT-5MR-700-15", "A-02 T1092 ST 20-065 AISLANTE", "VARILLA 1197/01-03-014", "4B211749-P0101-0 MAGNET HDDER - CW80", "10021975 DRIVER AND DRAIN SWITCH", "2961105 SINGLE RELAY REL-MR-24DC/21", "102-242-981 ASSY PCB WSX ERGO GUARD", "204-109 BEARING RAIL", "BES 516-3005-G-E5-C S49(BES00HF )", "MORDAZA #151202-L01M01U09", "FABRICACION DE SELLO #299H215214A", "WELD FLEXURE 4-32923-01", "Y5A50091 ENCODER, HEIGHT", "Y5A50095 SLIDE BEARING", "105-359 IKO RAIL #LRXG20C1R145T2HS2/HP", "204-049 FOLLOWER,CAM CYR-1-S", "205-254 CYLINDER,FABCO#FPS-903-17SK", "NOZZLE 2-1 201H094116", "NOZZLE 2-2 210H053319", "NOZZLE 299H170355", "PK569HNBW STEPPING MOTOR ORIENTAL", "CRK569HBPB STEPPING MOTOR UNIT", "PERNOS GUIAS #299H264137A", "NIDO ESCANEAR MA190", "PIN MA470_475_490_500", "CLAMP P1 MA470_475_490_500", "CLAMP 21 MA470_475_490_500", "BASE VERTICAL MA470_475_490_500", "BASE MA470_475_490_500", "WASS PLANTILLA DE URETANO 299H238416", "STOPPERT 299H235335", "BKT FIXTURA URETANO 299H249184", "STOPPERT 299H235430", "CLAW FIXTURA URETANO 299H236391B", "CLAW SUJETADOR DE BOTE 299H236256B", "CLAW SUJETADOR 299H240216A", "PIN PARA PALLET KFQSAPG6-P3.9-L6-B5", "299H201120", "299H236152B", "299H235329A", "299H180183", "299H249166", "299H236342B", "299H247167", "299H170385", "299H237325", "299H170386", "299H177325B", "299H235514", "299H240231A", "BKT-STOPER 299H249817", "BLOCK BASE PARA BOTE 299H183392", "299H182342B", "AIR GRIPPER MXS20-150B-A93", "CILINDRO PLANO MGPL12-100Z-A93", "CDM2RKB25-200Z-A93 CILINDRO CON SENSORES", "MXS12-100ASBT-A93L AIR SLIDE TABLE", "MHS4-50D-M9B GRIPPER CON SENSORES", "MSC-3B739842 P0 101-0 THIMBLE", "MSC-3B739843 P0 101-0 SHIELD", "MSC-2B739859 P0101-0 CENTER GUIDE", "STOPPERT FIXTURA DE PARO 299H235422", "299H173574", "MSC-4B739854 P0101-0 TONGUE GUIDE SLIDER", "MSC-4B739828 P0101-0 CORE PRESS", "HIWIN MGN9CC LINEAR GUIDEWAY", "COGNEX X-CODED M12 CCB-84901-2001-05", "MSC-4B739844 P0101-0 WORK CATCHER", "MSC-2B739858 P0101-0 CENTER GUIDE (TOP)", "MSC-3B739839 P0101-0 COLLECT CHUCK", "MSC-1B739835P0101-0 OUTER SHAFT", "SFC-035DA2-19B-12B COUPLING MIKI PULLEY", "CAUTIN HAKKO N/P 937-5 (FX-888)", "MRHQ20D-90S-N  ACTUADOR GIRATORIO", "79T9657 SPS-1820 POWER SUPPLY,BENCH", "EHSF1.5-160-P0.8-N69-HC2.9 EJECTOR PIN", "EHSF1.5-199-P0.8-N69-HC2.9 EJECTOR PIN", "EHSF1.5-163-P0.8-N69-HC2.9 EJECTOR PIN", "L93094-C5672 COLLET ( WINDER )", "L93095-C5679 COLLET", "FABRICACION DE INSERTO69 MOLDEO KN13100", "F96 FABRICACION DE GEAR F96", "MSC-4B739853 P0101-0 TONGUE GUIDE", "MSC-3B739920 P0101-0 WING A", "MSC-2B739852 P0101-0 CHUCK", "OP-87902 LENTE DE MAGNIFICACION", "PKS-399 302 250 A 4202 1 PNEUMATIC TEST", "E39-S63 SENSOR", "#541093 B05 BIT", "BES 516-3005-G-E4-C-S49-00,3 S INDUCTIVO", "SOLONOID VALVE 4GB229R-00-A2NH-3", "SENSOR PNP BES M08EE-PSC20B-S49G-003", "SENSOR BMF 303K-PS-C-2A-S49-00,2", "GRIPPER MHF2-12D2R-M9BL", "T.TRANSPARENTE  MT900179599", "JIG  299H214121B", "LAYERING  299H214122", "LAYERING  299H214123", "BLOCK  299H214198", "BLOCK  299H214399", "CONECTOR 3/8 X 3/8 NPT A 90", "RESORTE RC 01-020-374-190 PELE059 TS 06", "RESORTE RC 01-022-374-190 PELE059 TS 06", "VENTOSA TOP33906", "CENTER LOCATING INSULATOR 4228609", "SPRUE BUSHING HTR TC CLI 4190839", "NOZZLE HEATER 6996397", "THERMOCOUPLE 1502149", "RING CONNECTOR 2376509", "KEY BAR (BARRAS GUIAS) A840407900", "WORK HOLDER  299H215388", "GUIDE BLOCK 2  227H063519", "SPRING PIN  227H063439", "BLOCK 1  299H214235", "BLOCK 2  299H214236", "GUIDE 1  299H214241B", "GUIDE BLOCK 1  299H214244", "GUIDE BLOCK 2  299H214244A", "GUIDE BLOCK 3  299H214245A", "JIG 299H214269", "GUIDE BLOCK 4 299H214246", "CHUCK 299H214753A", "JOINT SHAFT ASSY 229H030433", "JIG 229H030413A", "STOPPER 229H030431", "PROBE BLOCK 229H030432", "CLAMP RUBBER 227H049231", "DIAMOND  V  BLOCK   N.P. DT-21693", "FU-59U SENSOR DE PHOTOELECTRIC", "BURIL KITZEL FF375-269", "BOMBA HIDR.PROCON  6XE94", "LOCTITE SF 7629 CONTACT CLEANER #1174633", "SENSOR EE-SX951-R 1M", "AIR CHUCK MHF2-16D1-M9BL", "AIR CHUCK MHZ2-16D-M9BL", "16108-01-00-179 VENTOSA", "LINEAR SHAFT SFJZ10-59-M6-N5-SC40", "SOPORTE DE MONTAJE E39-S64", "MT3290708 #90708 SOLID CARBIDE", "MT3290821 #90821 SOLID CARBIDE", "KN5310905 #10905 BALL-END HEX", "NAVAJA 4B297732", "09004581-SEAL KIT, OIL UNIT", "ORING 3.984 INTERIOR EN SERIE-200", "BALERO 7002A5TRDULP3 CD412910A Y 10B", "MAGNETICO SENSOR SMC D-M9PL", "3255984 NOZZLE TIP", "2325190 LOCATING INSULATOR", "7079771 WAVE SPRING", "3936720 FAHRENHEIT 800 BEARING G", "7298786 U750 UNH GEN2 REMOVAL TO", "7729746 VALVE STEM", "6965278 NOZZLE HEATER", "BELT #7099091A", "SERVO MOTOR VRDM3913/50LNB00", "3255989 NOZZLE TIP, P/F", "3731089 CYLINDER", "7122920 THERMOCOUPLE RING", "079340-97115 ELECTRIC ROTORSPRAY", "TIMUNG BELT 240L100 (ITEM NO:00694244", "L93983 3C DRAWBAR", "L93038 3C COLLET KEY", "MARKAL 96603 RS200", "HANDLE AP-197-1-3-IVORY", "#106397 SPACER RING", "MANGUERA NWP70-9-1350L (1004)=1004)", "EXTENSION APEX  M-490", "SY9320-5LZ-03 ELECTROVAVULA 5/3", "CY3R20-200-M9BL UNIDAD DESLIZANTE", "LINEAR ENCODER SYSTEM 9418", "TONER PLOTTER HP C4913A AMARILLO", "TONER PLOTTER HP C4911A CYAN", "TONER PLOTTER HP C4912A MAGENTA", "AIR REMOVAL INIT GUS1079-180930 POWER", "CONTROLLER 180931-1 POWER SUPPLY", "CLEANPOWER CMY-097 (18L/PAIL)", "CS95-63 KIT DE REPARACION", "CS95-80 KIT DE REPARACION", "CS95-100 KIT DE REPARACION", "CS96-125 KIT DE REPARACION", "CK95-63 KIT DE REPARACION PARA ANTIGIRO", "SPC046-M29 PORTA ELECTRODO SUPERIOR", "GREASE FILTER GF1420-6  KA10394A", "DISPESNE VALVE DV1003-LR   GPR7379", "GREASE PUMP GDP-400G60-NPN  9752", "CONTROLLER  180931-2   9417", "DISPENSER  AAPGD1178A-0.8-AR-EN2  9282", "RESERVOIR FGRA1250-A  8493", "CONTROLLER  180931-2  8058 WIHT 180931-2", "AIR REMOVAL UNIT GUS1079-180930 PLC WITH", "AIR REMOVAL UNIT GUS1079-180930 POLYPAK", "3B739197P0101-0 COLLET CHUCK", "AIR REMOVAL INIT GUS1079-180930", "AIR REMOVAL INIT GUS1079-180930 ANALOG", "CONTROLLER 180931-2 ANALOG INPUT CARD", "AIR REMOVAL INIT GUS1079-180930 O RING", "AIR REMOVAL INIT GUS1079-180930 SOLENOID", "AIR REMOVAL INIT GUS1079-180930 SENSOR", "AIR REMOVAL UNIT  GUS1079-180930", "GREASE PUMP GDP-400G60-NPN 9590 WITH", "CONTROLLER  180931-1  PLC WIHT PROGRAM", "CONTROLLER 180930 PLC WITH PROGRAMA", "AIR REMOVAL UNIT GUS1079-180930 ROD WIPE", "AIR REMOVAL UNIT GUS1079-180930 SLEEVE", "CRK569HBPB STEPPING MOTOR UNIT", "PK569HNBW STEPPING MOTOR ORIENTAL MOTOR", "CDQ2WB125-75DCMZ-A93L CYLINDER", "6147 FEED ROLLER (URETHANE)-M33,M93", "5459 SCREW ASSEMBLY", "3926 DOWEL PIN", "A-NID-ECMH-095", "AIR REMOVAL UNIT GUS1079-180930 HMI WITH", "CONTROLLER 180931-2 HMI WITH PROGRAM", "CONTROLLER 180931-1 HMI WITH PROGRAM", "CONTROLLER 180930 HMI WITH PROGRAM", "AIR REMOVAL UNIT GUS1079-180930 CYLINDER", "PULLEY MSC-4BH00948/698ZZ", "DRUM PULLEY ASSY MSC-3MK33975 B200S3M", "BOTELLA 4OZ PUNTA DE AGUJA 1902T128", "SPC047-M9  BUSHING ACERO", "ELEMENTO FILTRANTE 10 MICRAS #EHM19R10A", "CHUCK CLAWS 1809328", "KAPSTO GPN 240 MT 9.5 PROTECTIVE", "SENSOR EE-XX951-W 1M", "BIT 541093-B05", "SCREW GUIDE 1809327-B01", "TNR-HK0549, CABLE ASEEMBLY WITH BOLT", "BABDVV250953 BALA 25 VALVE BODY ( NS )", "09310425001 NISSEI GREASE NS1 700CC", "09009984-MOTOR ONLY FOR P# 09003669", "CDQ2A32-50DMZ-A93L CILIMDRO", "093104250-10 GREASE NS1 400CC YELLOW", "1769L32E COMPACTLOGIX 750KB ENET", "1769OB32 COMPACTLOGIX 32 PT 24VDC D/O", "PLASTIC WAND, 19 IN L, BLACK", "FABRICACION DE A-NID-ECMH-095", "CREVICE TOOL, 9\", 1-1/4\" HOSE N849", "DWG 4B739477  PARA MAQUINA AM030", "4MK02559-0-01E, NIPPER", "MBRVCP049092  SUPPORT PAD", "MIM18VV099-MASS 18 VALVE NOZZLE ASSEMBLY", "MFPTRI390100 - PIN GUIDE RING", "TNPGB0409CN0 TINA PIN GUIDEC BUSH", "CDQSFS20-30DC-A93, AIR CYLINDER", "1197/01-03-004", "9A9000700133.6  POWER CABLE 3.6M +2", "9A9000700033.6 RESOVER CABLE 3,6M + 2", "4GB239R-00-A2N-3 SOLENOID VALVE", "MORDAZA DE GRIPPER 3B203901", "1769L35E COMPECTLOGIX 1.5MB CONTROLLER", "1769OB32 COMPACTLOGIX 32 PT 24VDC D/O", "1769ECR COMPACTLOGIX RIGH END CAP", "1769PA2 COMPECTLOGIX AC 2A/0.8A POWER", "1769IQ32 COMPACTLOGIX 32 PT 24VDC D/I", "1769OB16 COMPECTLOGIX 16PT 24VDC D/O", "40160001  SEALING RING 10.9 / 7.4 X 1.43", "40 WELD 2 COIL SUBASSEMBLY SPC048-M9B", "00419051  VALVE PIN  2 X 203.29", "24M9335 ZB12-6 RELAY, OVERLOAD", "SA72G942A4 SA48-17-33BIT ENCODER", "CABLE DE CONEXION OP-87904", "FIXTURA 047-TIM-3920-TX-001", "PIN 299H264663A SUJ2", "NUT 299H264662A S45C", "JOINT JIG 299H264661D SUS440C", "2365-0951 ORIENTAL MOTOR", "C-G62952 BRUSH DRIVE FRAME", "1100-0922 BALL BEARING", "MESA GIRATORIA MSZA30AX-M9BL-X1", "C-G62951 ANGLE DRIVE BRACKET", "GDG-10745 CORE CENTERING   APA 3009-B", "SLIDE CHICO 471.016-209", "MDSUB20-90S-R80L  ACTUADOR GIRATORIO", "MHZ2-16D (MHB39)  GRIPPER", "GRC-5-90-T2H-D-A1  AIR CYLINDER (ROTARY)", "D-Y59AL  SENSOR NPN", "PUNTA TORX T25 6\" LARGO 7396A55", "1769L32E COMPACTLOGIX 750KB ENET", "8780A191 CARBIDE SQUARE-END FOUR FLUTE", "4179A236 LONG-LIFE BAND SAW BLADE", "8928A16 TICN COATED CARBIDE SQUARE-END", "4179A588 LONG-LIFE BAND SAW BLADE", "0046803 ARBOR 9", "GDG-10768 ARMATURE TEST PROBE AZS-100609", "0047693 TOOLING, SEPARATION, MCI761,OD", "6184  TIMING BELT 3MM, 96TH-M33", "A18006M-IBC-CLI093  COIL AOBA", "XOMD 03014-0902/01 CLAMP BLOCK", "R1666-194-20 B.RUNNER BLOKC CS", "COUPLING SFC-035DA2-16B-19B", "6906ZZ NSK DEEP GROVE BALL BEARINGS", "COUPLING SDWA-39C-14X16", "079340-984108 PISON WITH INTEGRAL ROD", "079340-984125-50 O-RING, BUNA N 50 PACK", "JIG #1 299H238225", "299H252919 CLIP", "299H252522 CLIP", "299H252521 CLIP", "299H252275  CHUCK I", "GRIPPER DE PIÑON #299H252522 DE LINEA", "299H252274  CHUCK R", "299H252273 FIXT CLIP", "A16011M-IBC-CL1O93 COL AOBA", "#AS568B-436 3BH02238+3BH02239+3BH0580X", "079340-984099 LOCTITE STROKE ADJUST MENT", "079340-984117 LOCTITE 984117 DIAPHRAGM", "3066A19 UNCOATED CARBIDE SQUARE-END MILL", "60S2M196GB TIMING BELT MITSUBISHI", "PIN 1  299H183387B", "PIN 2  299H183389B", "XOMD03014-9001 CONTER JIG CLAW", "TF 3007 M81 309 GRIPER EN DELRIN", "ACA1920-25GC SCAN CAMERA BASLER", "BMF0002  BMF 204K-PS-C-2A-SA2-S49-00,3", "SHPAHR20-L41-P7.97-B7 PIN GUIA PALLET", "P/N F49884 BRAKE SHOE-TOP ROLL", "P-670954 CERAMIC SUPER STONE RED", "21230 AS-9 1/4X1/4X6 100 GRIT", "21560 AS-9 1/4X1/4X6 180 GRIT", "P-669954 CERAMIC SUPER STONE GREEN", "34932 TH 1/4X1/2 150GRIT", "NSK-6009-2ZC3E BALERO 6900ZZ1C3E", "N1-19-146 PIN PALLET COMPLETO", "OP-30591 CABLE KI ( 20M )", "OP-86917 CABLE PARA SERIE VT", "7113K49 RING TERMINALS, VINYL INSULATED", "7113K98 RING TERMINALS, VINYL INSULATED", "WESP3-9-H15 SPROCKETS FOR CONVEYOR", "PIN GUIA NI-19-143 30MM DIAMAT COMPLETO", "PIN GUIA NI-19-144 30MM DIAMAT COMPLETO", "A16011M-IBC-CLI093 COIL  (FOR IBC#1)", "G2 STOPPER-2 X0M03014-9015/01", "L93986-3C SPINDLE", "196150 MHE2-M1H-3/20-M7", "HK-03-061-009 PLACA SISTEMA DE ASPIRADO", "RESORTE DE COMPRECION ESPESOR 0.9MM", "NV-NF7H9CLV-G04-AB HEATING COIL", "SIM-19-335 SELLO FUGA DE AIRE DE URETANO", "CP96SDB63-50C CILINDRO NEUMATICO 163X50", "CP96SDB63-150C CILINDRO NEUMATICO 63X150", "CP96SDB80-160W CILINDRO NEUMATICO 80X160", "CP96SDB100-200C CILINDRO NEUMATICO", "CP96SDB125-200 CILINDRO NEUAMTICO", "0089007 KIT,SPARE PARTS,POWER SUPPLY", "SCSA90490140F0 POWER MODULE FOR A90 BOX", "AFH-A22-02123 GUIDE STRIP 5.5 X 35 X 96", "0051795 SEAL TOOLING  APPLICATION SET", "539158 ELECTROVALVULA VSVA-BM52-AZD-A1-", "539156 ELECTROVALVULA VSVA-B-B52-ZD-A1-", "299H253218 FIX BLOCK", "299H259715 PLATE", "299H263283 JIG", "299H261516A WORK PLATE", "299H262212 SEAL PLATE", "299H261212A JIG", "MGN9HH BLOQUE LINEAL", "B-93702-8  GLOBE CYLINDER", "C-L93015-1MOTOR MOUNT URI ROTATOR", "1492SPM1C040 MCB SUPPLEMENTARY PROTECTOR", "100C09EJ10   IEC 9 A CONTACTOR", "BANDA 309-3M-19", "299H260333B BRACE", "0024589 MOTOR,CONVEYOR,3X220/480V,50-60", "0030976 VALVE,AIR,24VC,EVP542-5YOB-03FA", "0045749 VALVE BANK,COMPLETE (M761)", "97-010-01 TORCH BODY MB0712072 TA 200SSP", "INSULATOR MB0309056TA-23A", "0051795 TO SEAL 1823111-1 VERSION 3A RED", "K005-7890 AKD-P01207-NBEI-0000 SERVO", "1100-0879 BEARING", "1175-0396 COUOLING", "1900-0370 AIR COOLED CABLE", "299H257215 SUPPORT BASE", "ACEITE  LUBRICACION OFSW-32 152811 DM896", "CONECTOR ELECTRICO EPIC 10.1960", "GUANTE DE NITRILO  FRT9337L", "CEPILLO DE ALAMBRE 254-B-954014", "CANDADO N/P 98410A-128", "PILA ALKALINA 9V CUADRADA", "9SM2002B000000 VIBRATION TRANSDUCER", "SPR-4B03927800P0101-0 SPRING", "LARGE NOZZLE TIP-O RING .395 ID X .040W.", "FIBRA VERDE 3M USO GENERAL P-96", "LIJA FANDELI A-99  400", "CODO 1/8 NPT X 1/4 POLI #169-PLNS-4", "GUANTE TIPO HYFLEX  KEVLAR,FRKEV43169", "LOCTITE BOTE 10ML 262  #26221 (DM-849)", "O-RING .989 ID X .070 W 2-022 70", "BANDA 1/2 ANCHO X 39 LARGO", "BASE RELEY #27E894", "CABLE CONECTOR ANGULO 159420", "SENSOR SMC D-A93L", "GUANTE ALTA TEMP. 89307961", "1773951 A00 SCREW GUIDE HOLDER ASSEMLY", "C42D17FK7D MOTOR 3/4 HP 098032.00", "MANOMETRO # 162839-MA5016 1/4", "\"V\" SUPPERIOR #3BMKX31A009000", "SENSOR INDUCTIVO M08X1 NPN (BES00C9)", "GEARMOTOR TYP 24A4BEPM-D3 MODEL#0189", "GOMA A-02T1108ST30-009", "299H259713 BRACE 2", "299H263264B JIG 1", "299H263711 JIG 1", "299H263712 JIG 2", "299H262246 UPPER PUSHER PAD", "299H260243A CARRIGAE", "1.50J2HHNAT1S29A7.000 CYLINDER PH GEN 2", "BARRENO PILOTO DE 1/4' (1.809') PASO25", "16107-01-03-19 DERECHA GUIA NIDO", "PUMP.SEAL KIT #0900358", "4MF34029-0-01E FELT PAD", "BALL NUTS NOOK IND.SBN-9578 035-0125RH", "299H261934A BLOCK CHUCK", "PISTON BELOFRAM 980-077-000)", "HOLD PLATE 299H261557A", "16107-01-03-19 GUIA IZQUIERDA NIDO", "HAKKO ESD IRON MEDIUM 907 N/P C1148", "BES M08EE-PSC15B-S49G-003 S INDUCTIVO M8", "SHEET 299H253320", "HOLD PLATE 299H261558", "CODO 1/4 NPT X 3/8 # 169 PLNS-6-4", "C9225H24BPLB-W-7 FAN", "RLAY 17M9929 KRPA-14DG- 24", "VALVULA APLIC. GRACO 224906", "PUNTA P/DES.TORX APEX 49-C-TX-20", "299H253412 SEAL PLATE", "M-N-852790 ALLEN BRADLEY PANEL VIEW", "SLOT SENSOR DIAMETER 4MM  9CSADPS26BAE90", "3842515492 POLEA DENTADA", "3842218920 COPLE MACHO A HEMBRA", "3842218921 CLUTCH MACHO A MACHO", "GRC-30-90-T2H3-D AIR CYLINDER (ROTARY)", "B6902ZZ DEEP GROOVE BALL BEARINGS", "B6901ZZ DEEP GROOVE BALL BEARINGS", "RODILLO DE RETORNO B Y PERNO D=19.6X26", "01M-972-01-1-7-1", "TOLOMATIC 01090000 LEFT HAND 2 WEEKS", "1.50J2HLTS29A7.00 CILINDRO HIDRAULICO", "BGSYB6906ZZ-35 DBL BEARINGS & HOUSING", "MHPUS408-50-19-A CABLE CARRIER", "JBPE20-P18.0-W12.0-L9 PIN BUSHING OVAL", "CABLE/SENSOR ANGULO P/N 159422", "HHB6902ZZ BALL BEARING", "B6903ZZ DEEP GROOVE BALL BEARINGS", "STP-MTRH-23079 SURESTEP STEPPER MOTOR", "C-B6900ZZ BALL BEARINGS", "UNV20962 CARPETA VIEW 11X8.5 .1\" BLANCA", "UNV20982 BNDR VIEW 11X8.5 .2\" WE", "SAM16797 CARPETA BLANCA DE 4\"", "UTSMA5-29-15 URETHANE SHEET", "B7009SU BALL BEARING", "CODO1/4NPTX1/4 #169-PLNS-4-4", "4B359802 HUSILLO DE HERRAMENTAL LADO (A)", "4B359803 HUSILLO DE HERRAMENTAL LADO (B)", "4B359807 HUSILLO DE HERRAMENTAL LADO (A)", "4B359808 HUSILLO DE HERRAMENTAL LADO (B)", "4797A11 BRUSH WITH SHANK FOR ANGLE", "4911A17 BRUSH WITH SHANK FOR TIGHT", "B7009-E-2RSD-T-P4S RODAMIENTO DE", "SIM-19-1328 BOTTOM PRESS 1", "SIM-19-1329 BOTTOM PRESS 2", "CT-5239 TARJETA NATIONAL MODELO NI-9234", "NI-19-218 GUIA PARA RUTEO BUSBAR", "3B359799 HERRAMENTAL DE BOBINADO LAD (B)", "3B359798 HERRAMENTAL DE BOBINADO LAD (A)", "FL6902ZZ BALL BEARING", "RV3D20-90-45-SR-U AIR CYLINDER (ROTARY)", "CMK2-C-LB-25-290-T2H3-D AIR CYLINDER", "RELEY 36X1970MAGNECR.750XCXM4L-120A", "P/N 90B8644 FIBER OPTIC BEAM#E32-T14L", "MCLPTK6-1 COUPLING FOR TUBE-90 DEG ELBOW", "HE-G3/8-LO VALV. DE SEGURIDAD IND.197133", "SAN39100 MARCADOR SHARPIE SR COLOR PLATA", "609-2RS SLB ROD. BOLAS MINIATURAS C/TAPA", "NOZZLE TIP .499 DIA X .934 440 C", "DWG19-723-100 BASE PARA COLOCAR BANDERA", "DWG19-703-102 PERNO GUIA", "DWG19-723-105 PERNO PORTA BANDARE", "SE2B16-190 SLIDE GUIDE", "SGD7S-R90A30AYASKAWA S7S AMP100W 200V", "BEARING BALL N/P N-872898", "GRC-5-90-T2H-D-A2 AIR CYLINDER (ROTARY)", "GRASA LUB.ALT.TEMP. #LO161-098 (DM 279)", "MOTOR PINTTMAN GM9213-4", "299H236298 CLAW EN MATERIAL URETANO 90A", "X0MD03001-0901_03/CLASS FIXTURE SHELL", "D1MD03001-D023_03_150109/CLASS JIG", "USP590-1U2 AC SPEED CONTOLLER", "BALL PLUNGER 1/4-20X1/2 #10905", "VALVULA DE ARRANQUE HEL-D-MIDI 170691", "CILINDRO TANDEM DNCT-80-100-PPV-A 191110", "VALVULA DE ARRANQUE HEE-D-MIDI-24 172959", "CDU20-10D-A93 PISTON", "779593-01 NI 9239, MODULO DE ENTRADA", "779760-01 NI PXI-1033 CHASIS, MXI EXPRES", "BK9000 ETHERNET COUPLER", "80K9315 SDN10-24-100P AC- DC CONVERTER", "40M7849 SDN 5-24-100C AC/DC CONVERTER", "DWG19-803-101 FLECHA PARA CONVEYOR", "DWG19-803-104 FLECHA PARA ENGRANE", "DWG19-803-105 ENGRANE PARA CONVEYOR", "KBIC-125(9433L) CONTROL DE VELOCIDAD", "K93049 MDF8500 FLIER HUB", "3SBM406G900170 INSERT FOR GRIPPER", "DWG19-824-107 FIXTURA PARA COLOCAR BRUSH", "DGW19-824-106 FIXTURA PARA PEGAMENTO", "DWG19-824-113 FIXTURA PRENSA DE LIGA", "DWG19-824-114 FIXTURA PRUEBA HIGHT SPOT", "DWG19-824-118 FIXTURA GUIAS DE PALLET", "DWG19-824-121 FIXTURA SOSTENER MOTOR", "DWG19-824-122 PALANCA ESTACION M120", "DWG19-824-123 PERNO PARA TOPE", "DWG19-824-124 PERNO PORTA RESORTE", "DWG19-824-125 PERNO GUIA", "DWG19-824-126 SHOCK ABSORBED PARA PISTON", "CDAQ-9178 (8 RANURAS USB)", "DWG19-824-100 FIXTURA COLOCAR NUCLEO", "DWG19-824-101 FIXTURA INSERTAR FLECHA", "DWG19-824-103 FIXTURA COLOCAR ARMADURA", "DWG19-824-104 FIXTURA COLOCAR BRUSH", "DWG19-824-105 FIXTURA COLOCAR BRUSH", "DWG19-824-108 FIXTURA DETECTAR BRUSH", "DWG19-824-109 FIXTURA PRENSADO DE CABLE", "DWG19-824-110 FIXTURA PRENSADO DE CAJA", "DWG19-824-111 FIXTURA SOLDADO DE TERMINA", "DWG19-824-112 FIXTURA PRUEBA ELECTRICA", "DWG19-824-115 FIXTURA PRUEBA DE FUGA", "DWG19-824-116 FIXTURA PRUEBA PERFORMANCE", "DWG19-824-117 FIXTURA BASE DE SENSOR", "DWG19-824-119 FIXTURA DERECHA DE GRIPPER", "DWG19-824-120 FIXTURA IZQUIERDA GRIPPER", "362050 SRU+35-W-180-90 GRIPPER SCHUNK", "4PK975 BANDA SERPENTINA", "CY3R25-100-M9BL PISTON", "CDU20-20D-A93 PISTON", "CDG1LN20-100Z-M9BL PISTON", "MSQB20L3-A93L PISTON ROTATORIO", "2365-0952 GEAR MOTOR (51K40A-AW2)", "MY1H20G-350L7-M9BL PISTON", "B.BRUSH 13\" LONGTH 1\" TRIM LONGT #100973", "209H040148A CUSHION", "209H040134A UNDER", "TDC-1009 POWER SUPPLY, INVERTER DC", "103H8221-0941 SERVO", "TYPE 48Y6BFPP 3842503590 MOTOR", "TYPE 34Y6BFPP 8981001818 MOTOR", "M2E052-BF88-59 MOTOR", "SGMGV-09ADA21 SERVO MOTOR YASKAWA", "VRGF-20D120-19DC19 SPEED REDUCER SHIMPO", "PIEZA#16008-1-09-07 EN MATERIAL ACERO A2", "FABRICACION DE SHEET 299H265128A", "LAYERING 209H040135A", "079340-97233 LOCTITE 97233 EQUIP LUER", "JIG 209H040185 FABRICACION DE PRESS", "JIG 2 299H264369 FABRICACION", "PUSHER 299H265142 FABRICACION", "JIG 1 299H264368 FABRICACION", "JIG 299H264356A FABRICACION", "POGO PINS  # LS093R-618-N-5.4", "FIXTURA PARA SOLADAR BRUSH DWG19-843-103", "GUANTES ANSELL 11510 TALLA 9", "2901 DEREEL PULLEY 45MM YUASA", "202-319 DEREEL WIRE CLEANER CLIP", "50997 SPRING COMP .420 OD 2.00", "50569 SPRING EXT .625 OD 3.00 L", "50572 OE DREEL DANCER ARMS 6MM,1MM,900MM", "2913 BELT 51T 255MM PL 10MM W CHUCK STAB", "52538 SHLD-SCR 5MM X 29MM LG, TOP ROLLER", "4979 BA-BRG 5MM 13MM 4MM", "PUNTA DE PRUEBA MODELO: 912-312R", "RF2080S912T SPROCKET", "6FCD10 J0=F7737 6609070-1", "GLOBE PN 116957 INPUT FIELD TERMINATION", "GLOBE PN 116953 4 AXIS QUADRATURE BREAKO", "93014-21 WHOLE ASSEMBLY", "BL 93037 COLLECT KEY", "BK-93254-7", "BK 93440-C4509", "C K 93255-1", "K93124-1", "3M059D DAYTON MOTOR", "299H266115 BLOCK", "299H264214 GUIDE", "299H267113A JIG", "299H271377 FIXTURE PLATE", "299H271338A GUIDE", "299H271355 FIXTURE SEAT", "299H271354 CLAMPS 3", "299H271341A JIG", "299H271353 CLAMPS 2", "299H271352 CLAMPS", "299H271339 GUIDE 2", "299H264213 JIG", "299H266216A CLAMP RUBBER", "PSFJW8-29-M5-N5 LINEAR SHAFT", "MATAA8-P7.97-B5.0-T10 LOCATING PIN", "299H267124 JIG", "299H266231 PROBE HOLDER", "299H266232 HOLDER", "299H267125 BLOCK", "0234-3M-9 (AM040) BANDA DE TIEMPO", "0279-3M-9 (AM040) BANDA DE TIEMPO", "DWG19-843-101 HOUSING PARA TRACCION", "SHPAHR20-L30-P7.97-B5 SUPPORT PINS", "SDPAHR20-L30-P7.97-B5 SUPPORT PINS", "LPGGA6-P8.00-B18.0-R6-L9 LOCATING PIN", "DWG19-843-102 ADAPTADOR PARA HOUSING", "299H261158A ELECTRODO COBRE NIQUELADO", "299H270162A ELECTRODE 2", "93222-C5672 R GUIA DE AMARRE", "C K 932223-C5105L", "C K 93223-C5105R", "C K 93222-C5672-L", "93032-6", "299H270163A ELECTRODE 3", "299H270159 STOP PLATE C", "299H270157 STOP PLATE A", "299H264212", "299H270158 STOP PLATE B", "299H270161A ELECTRODE", "SDNR21-01-009 FIXTURA", "PICK OFF PINS  #329406 (JUEGO)", "TF3252-20-719-02 TORCH MOUNT", "A-02 T1092 ST 20-008 NIDO A", "72-2690, TENMA BENCH POWER SUPPLY", "UPCN19-B-36 PULL", "DWG19-843-100 FLECHA PARA TRACCION", "GP-OPT2-9 OPTICAL RS-232C MODULE", "CP96KDB63-200C CILINDRO NEUMATICO", "CP96SDB63-125C CILINDRO NEUMATICO", "123093006 LAMP 110VAC 55W", "I/O MODULE,DR-ODC5 #96FI873", "PAWS 1 16108-01-00-091", "595-1014-ND XFRMR LAMINATED 10VA THRU", "299H271350 SOCKET", "299H266219 STOPPER", "299H264816A CHUCK", "299H266221 SPRING STOPPER", "SDPAHR20-L41-P7.97-B5 SUPPORT PINS", "MATDA8-P7.97-B5.0-T10 LOCATING PIN", "PRC04-12A20S-19M14.5 CONNECTOR", "CLAW 203H165521A MC901", "1350-2560 FS-09-6.062-BMMTW BIMBA", "B-G62920-8 CYLINDER COUPLER", "1350-2563 D-5379 CYLINDER NUT", "G62953 BRUSH ADAPTER SHAFT", "BG62945 ROTARY ACTUATOR MOUNT", "B G62945-1 ROTARY ACTUATOR MOUNT", "MY1H25G-450L-M9BL", "MY1H25G-350L6Z-M9BL", "MY1B40G-250LZ-A93L CYLINDER", "RSDQB16-15D-M9BL AIR CYLINDER", "PRC04-21A20S-19F CONNECTOR", "D039_01  D039_01 CLASS 2.8 PALLET", "BIMBA CYLINDER  PFC-093-P", "B G62936 STOP PLATE COLLAR", "1450-2190 12750-4C-4B SHOULDER SCREW", "B250S5M390GB TIMING BELT MITSUBOSHI", "2330895 NYLON-12 TUBING SEMI-RIGID", "MXS25L-150B-A93L AIR SLIDE TABLE WITH", "MY2H25G-300L-A93L RODLESS CYLINDER", "HFSQN4-1540-594 ALUMINUM FRAME", "URETHANE PLATE 299H265121", "JIG 299H265114A", "B6905ZZ DEEP GROOVE BALL BEARINGS", "RORLM30-12-LC90 PIPE ROLLERS", "SLSBWF14-98 HEX POSTS", "HTBN279S3M-100 BELT", "299H241114 PLATE", "299H241115 DOWN PLATE", "SENSOR BKT 299H249818A", "299H183387C PIN 1", "SDNR21-09-024 CHUCKB", "299H271356 FIXTURE SEAT 2", "299H266213 JIG", "MHPUS102-19-13-S CABLE CARRIER", "299H264823A BLOCKBLOCK", "FPBTA6-P8.00-L9-B6.0 LOCATING PIN", "299H271357 FIXTURE SEAT 3", "299H269117A BLOCK", "GDMSB5.5-10-F9-M5 SHOULDER BOLTS", "MRS232-09M4N-09F-2 RS232C CABLE", "299H264367 STOPPERS", "BNR18D08-AMY009-P017", "BNR18D08-AMY009-P015", "BNR18D08-AMY009-P016", "BNR16G08-AMJ003-01-P009", "POGO PIN GUN PKS 399204200R42021", "ME-14011 AGF 0209-A RUBBER DIPRHRAGM", "MGN12C1R95ZAC BLOCK & RAIL 95 MM E=10", "AAA-S22-92000 DRIVE-CORNER", "AAA-S22-92300 DRIVE-250MM, ORIENTAL", "YT18-036-260-1-2009 ELECTRODOS", "RF2040VRPA-198L DOUBLE-PITCH CONVEYOR", "SF90E MOTOR CONTROLLER", "90YT120GV22 MOTOR", "61901-2RS AMB RODAMIENTO DE BOLAS", "299H266214 GUIDE PIN", "299H266218 PROBE BLOCK", "299H271337 CUSHION", "299H269112 JIG", "299H271344 DUIDE PIN", "299H271346A CLAMP RUBBER", "DC109 COMPRESSION SPRINGS", "DC099 COMPRESSION SPRINGS", "AL-39DF ALIF SENSOR", "SCXW46-12-19 COUPLING-HIGH RIGIDITY DISC", "MDSUA7-90S CILINDERS PNEUMATICS", "90GF10H GEAR HEAD", "90YT90GV22 MOTOR", "SWS31-90 COIL SPRING", "R16-5T3-FSIFW-119-160-0.05 HIWIN", "BNR16101-AMJ006-P019-1 PIN GUIA", "SFT1290-20-C MANGUERA DE TEFLON 12MM", "MGW9HZ0H LONG BLOCK 9MM HIWIN", "3-842-311-949 BLOCK CYLINDER", "RA9008CUUC0 CROSS ROLLER RING", "1837389B24 BIT COVER", "EE-SX952-R 3M F-SHP 5MM PW NPN", "EE-SX953-R 3M R-SHP 5MM PW NPN", "EE-SX954-R 3M U-SHP 5MM PW NPN", "MGN-09-C-1R005-Z0-H-M", "MGN-09-H-1R0055-ZF-H-M+U", "MGN-9-C-R0430-ZF-H-M", "MGN-09-C-3R0430-ZF-H-M", "MGN-09-C-9R0795-ZF-H-M+U", "328996 RODILLO DE REGRESO", "DVUS990W1 SPEED CONTROLLER PANASONIC", "BOS Q08M-PSLE20-S49 BARRERA", "BNR16G08-BMS009-P010 SHAFT POSITIONG PIN", "299H261157A BLOCK", "299H261911B BLOCK CHUCK", "O-RING BACK-UP 8-112 N300-90", "RUNNER PULLER, 4591 GEAR HOUSING D2", "PORRON SCALE CLEANER 20 LT ADESA  DM-957", "BUSHING INSERT S-MOTOR KN15092R1-PC2-014", "BUSHING INSERT S-MOTOR KN15092R1-PC1-014", "BNR16G08-BMS009-P001", "BNR16G08-AMJ002-P019", "BNR17I01-AMM009-P020 SCREW BIT", "BNR17I01-AMM009-P024", "BNR16G08-BMS009-P002", "BNR16G08-BMS009-P009", "BNR16G08-BMS009-P018", "BNR16I01-AMJ007-P029 CENTERING PIN", "4-32169-02 ELECTRODE BLOCK RIGH SIDE", "4-32169-01 ELECTRODE BLOCK LEFT SIDE", "JAW PUSHER (TZ054-593)", "BNR16G08-BMS009-P017 PIEZA EN URETANO", "563912 KIT REPAIR MSA-10", "187590 RETAINER", "05319GS06407 ZEBRA WAX RIBBON 64MMX74M", "299H264636B PIN GUIA", "SPACER TF3007M-81-619", "GRIPPER TF3007M-81-309", "TF3007M81-009 ROTOR HOLDER", "TF3007L-77-239 CHUCK", "TF3007L-79-136 CENTER PIN", "TF3007M-81-219 PIN", "TF3007-79-009-01 FINGER", "TF3007-79-128 PUSHER", "TF3007J-61-009-01 HOUSING SITTING JIG", "TF3007-79-114 PUSHER", "TF3007-79-007-01 FINGER", "TF3007-79-120 PIN", "TF3007-79-008-01 FINGER", "4289A27 PORTADRO DE NAVAJA C42", "BANDA MEGADYNE JASON B49", "R1666-194-21 WKD-015-SKS-C0-N-1 BLOCK", "698ZZ/5K NTN", "EE-SX952-W 3M PHOTO MICRO SENSOR", "TF3007C-12-309 TABLE JIG", "SFC-035DA2-9B-12B COUPLING", "CUSHION DWG: 299H260697", "FINGER DWG: TF3007B-11-01901", "299H260674 POSITIONING BLOCK", "299H260632 BRACE 1", "299H260686B CUSHION", "299H260633B BRACE", "TF3007B-11-02900 FINGER", "TF3007K-67-619 ROUGH GUIDE", "TF3007C-14-914 CLAW", "TF3007G-41-309 PULLING SHAFT", "TF3007L-79-024 JIG", "TF3007L-79-121 PABLE JIG", "TF3007M-81-509 PRESS HEAD", "TF3007-79-119-01 JIG", "TF3007-79-105-01 PUNCH HEAD", "SSR25XW4UU+1960L LINEAR GUIDE", "2H592 MOTORREDUCTOR CD,L 14-3/8 PULG,90V", "TF3007C-14-933-1 FINGER", "5331-05-000-0450 10259098B3187 POLYURETH", "EE-SX-974C1 SENSOR DE OVERTRAVEL", "8099 KSC WIRE SPRING DS", "JZCP-CS19-2-E CONNECTOR KIT", "FINGER B TF3007C-12-419", "TF3007K-67-709 SHAFT", "DIE SPRING, RED 9-1212-26 HEAVY LOAD", "299H262217 LOCATING BLOCK 3", "299H262218 LOCATING BLOCK 4", "299H262216 LOCATING BLOCK 2", "299H262215 LOCATING BLOCK 1", "299H261138 GUIDE 2", "299H261137 GUIDE 1", "299H261136A JIG 2", "299H261135A JIG 1", "299H262219 COMPACTS BLOCK", "#4-3B681349P0101 GRIPPER PARA SUJECION", "MGN9CZ0H MGN-9 BLOCK", "QHW20CA2R2920C+22 LINEAR GUIDEWAYS", "MGPM32-250Z-A93L COMPACT GUIDE CYLINDER", "MHS3-50D-M9BWL 3 FINGER GRIPPER WITH", "BNR 19D08-DMD008-A002-P055", "299H254223 LOCATING BLOCK", "299H263717 LOCATING BLOCK 3", "299H263716 LOCATING BLOCK 2", "299H263291 LOCATING BLOCK 3", "299H263289 LOCATING BLOCK 1", "299H263132 PRESS GUIDE", "299H263715 LOCATING BLOCK 1", "FU-59 FIBER UNIT THRUBEAM", "MGH-15-H-4R1590-Z1-H-M", "MGPL16-40Z-A93L COMPACT GUIDE CYLINDER", "299H265121B URETHANE PLATE", "RB500-SSC6-PG39 PRESSURE REGULATOR WITH", "CLAMP BLOCK 2 SDNR21-10-079", "CHUCK RUBBER A SDNR21-09-027", "354.519 LOCK RING SB30", "812.008 R-59 TOOL HOLDER", "4BS26549P0101-0,PLATE 2 GUIA NAVAJA", "4B191622 P0101-0 FELT", "299H267121 JOINT SHAFT", "97-010-01 COLETTE CHUCK 2.4 MB0507141-24", "97-010-01 COLETTE 2.4 MB0507142-24", "251H005249 STOPPER (CUÑA)", "299H266116A STOPPER", "299H266114 JIG", "299H265137 JIG", "299H264357A PIN", "209H040165 PROBE", "299H264335 JAWS", "209H040187 PRESS JIG", "MGPM32-50Z-A93L CYLINDER", "001 RSAO 1+3/16 PIL BLK 00560898", "165894 POWERPACKAGE K 4.300.20-US", "WAS-TU 959 ACERO HERRAMIENTA VARILA H-13", "MRS232-09F-09F-CROSS-3 RS232C CABLE", "U09A-AF-AM-0.5 USB CABLE", "FENM50-A985-B660 FENCE NETS - WELDED", "FENM50-A985-B525 FENCE NETS - WELDED", "FENM50-A985-B325 FENCE NETS - WELDED", "FENM50-A985-B555 FENCE NETS - WELDED", "FENM50-A953-B596 FENCE NETS - WELDED", "FENM50-A953-B371 FENCE NETS - WELDED", "FENM50-A925-B300 FENCE NETS - WELDED", "SS5Y5-41-09-C6 MANIFOLD", "GEAR HEAD 90GF5H", "CONECTOR ELECTRICO EPIC 10.1970", "93.693 PACKING RING D=22/30", "ANGLE PIN LOWER SMOTOR GEAR HOUSING 4591", "299H254322B LOCATING BLOCK", "299H257219 LOCATING BLOCK 4", "299H263290 LOCATING BLOCK 2", "299H263713 GUIDE 1", "299H259729 ARM PLATE", "299H254224 LOCATING BLOCK", "299H261175A PRESS", "299H263714 GUIDE 2", "299H263719 WORK PLATE", "299H260253 PALLETS", "299H257220 LOCATING BLOCK 3", "299H263292 LOCATING BLOCK 4", "299H263718 LOCATING BLOCK 4", "299H261174A PRESS BLOCK", "299H253217 SEAL PLATE", "299H259719 PROBE PLATE", "299H263265 JIG 2", "299H261118A JIG", "299H254212 LABEL JIG", "299H153788 BRIQUETTING", "299H257218 LOCATING BLOCK 1", "229H030431 STOPPER", "299H263239 JIG", "299H263266A JIG 3", "299H254225 LOCATING BLOCK", "299H263267B JIG 4", "299H254321A ADSORB JIG", "299H261178 ELECTRODE", "299H254222 LOCATING BLOCK", "299H258232 BLOCK", "299H259712 BRACE 1", "B696ZZ DEEP GROOVE BALL BEARINGS", "6900ZZ NSK DEEP GROOVE BALL BEARINGS", "MPW-01-2-40 29 PSI MODULAR PILOT CHECK", "OP-87906(IX) I/O CABLE FOR IX SERIES (3M", "CCMT09T304NE-KPD001 KYR TURNING TOOLS", "A16Q-SCLCL09-18AE KYR MILLING HOLDERS", "A16Q-SCLCR09-18AE KYR MILLING HOLDERS", "A12M-SCLPL09-16AE KYR MILLING HOLDERS", "VP-LDS-6X90 OSG END MILL", "CPMH090308NE-KPD001 KYR TURNING TOOLS", "TF3007A-05-029-00 CLAMP BLOCK2", "3842503069 GEAR REDUCER", "TAP CONE 2.35X6.95X0.5X0.375 (245)", "1890 ESCOBA ABANICO LARGA", "336 MOTA MECHUDO 90 CM PROFESIONAL 6403", "330 BASE MECHUDO 90 CM.", "GB-K 309L-16 1/8 KILO DE ELECTRODO PARA", "NITROGENO T 9 MTS  DMZ13", "ARGON ULTRA ALTA PUREZA99.999", "9155T51 COTTON TERRY HEAT 9-1/2\" LONG", "CCMT09T304NE-KPD001 KYR TURMING TOOLS", "CLAW HOOK 4B203995 P0101-0", "CLAW(2) 4B674496 P0101-0", "LOCATOR BLOCK 4B617937 P0101-0", "XOMD03014-9013/01 GZ-LIMIT FLANGE", "BNR19B08-AMG022-P015", "BNR19B08-AMG020-P024", "BNR19B08-AMG022-P016", "BNR19B08-CMY004-P034", "BNR19B08-DMD002-A002-P022", "BNR19B08-AMG011-P011", "BNR19B08-AMG021-P012", "BNR19B08-DMD006-A000-P004", "BNR19B08-AMG008-P055", "BNR19B08-AMG007-P007", "BNR19B08-DMD007-A000-P020", "BNR19B08-DMD010-A002-P013", "BNR19B08-AMG021-P013", "BNR19B08-AMG026-P031", "BNR19B08-CMY002-P017", "BNR19B08-CMY006-P091", "BNR19B08-AMG011-P026", "BNR19B08-CMY006-P062", "BNR19B08-AMG013-P009", "BNR19B08 - AMG008 - P056", "BNR19B08-CMY10-P003", "BNR19B08-DMD002-A001-P009", "BNR19B08-AMG003-P016", "BNR19B08-AMG007-P001", "BNR19B08-AMG004-P009", "BNR19B08-DMD001-A004-P011", "BNR19B08-AMG016-P014", "BNR19B08-CMY006-P073", "299H477332 URETHANE SHEET", "BNR19B08-AMG007-P006", "BNR19B08-AMG013-P010", "BNR19B08-AMG003-P062", "BNR19B08-DMD001-A003-P014", "BNR19B08-CMY010-P010", "BNR19B08-DMD001-A003-P010", "BNR19B08-CMY006-P090", "BNR19B08-DMD010-A001-P008", "BNR19B08-DMD009-A002-P044", "BNR19B08-DMD002-A002-P031", "BNR19B08-CMY006-P089", "BNR19B08-DMD001-A003-P033 BASE PARA NIDO", "BNR19B08-DMD001-A003-P013 PIN GUIA", "BNR19B08-DMD003-A000-P005 BASE", "BNR19B08-DMD004-A000-P008 BASE", "BNR19B08-DMD007-A000-P006 NIDO", "BNR19B08-DMD007-A000-P014 BASE", "BNR19B08-DMD008-A002-P038", "BNR19B08-DMD009-A002-P038", "BNR19B08-CMY010-P009 PALLET ROTOR", "BNR19D08-DMD002-A003-P006 BASE TUERCA", "BNR19B08-CMY003-P005", "BNR19B08-DMD004-A000-P010 CRIMPEADO", "BNR19B08-AMG003-P017", "BNR19B08-CMY004-P013 PIN GUIA", "4B865499 GUIA PARA FIXTURAS DE CENTRADO", "BNR19B08-DMD002-A003-P013 SELLO DE VACIO", "KFQSAGH3-P2.97-L5-B4 LOCATING PIN", "BNR19B08-CMY006-P089 YORK PALLET CARGA", "X0MD03014-9024, GZ -BASE PLATE", "TUBO HIDRAULICO 3/8 X 0.49 DE PARED", "ALF-MJ251975 BROCA HSS 5.00 MM (0.197\")", "G-90890200794 BROCA HSS 5/16", "TIS-5-161-133 BROCA HSS 6.60 MM (0.259\")", "10N49 BOQUILLA ALUMINADA 5/16 #5", "XOMD03014-9030/01 GZ-FIXED BLOCK", "XOMD03014-9004/01 POSITIONING BLOCK", "XOMD03014-9003/01 SUPPORTING SEAT", "XOMD03014-9031/01 GZ-HIT HEAD", "XOMD03014-9007/01 GZ-ADJUST SCREW", "XOMD03014-9020/01 GZ-PULL THE HEAD N", "SB612967 LIMA CUADRADA BASTARDA 6'", "TRUPER-15169 LIMA MEDIA CAÑA, BASTARDA,6", "C4-390.410-50 080A HSK TO COROMANT CAPTO", "ALPX2.9 FUNDENTE PARA ALUMINIO", "HEWC2P23AN INKCART HP 934XL HY BK", "SELENOIDE VALVE #09001551", "CARTRIDGE SP2003271 5TTR11NX-060029", "CARTRIDGE UFP-0695LH 5BXR16NX-060656", "L40920 145 RMP40 - RADIO/RADIO RENISHAW", "L40920 42 BREAK STEM KIT FOR M RENISHAW", "STFCR 08CA-09 CORO TURN 107 CARTRIDGE", "5BSR11NX-054892_TB01_00 BORING BAR", "C4-391.14-20 052 COROMANT CAPTO ER COLLE", "TCMW090204FP CORO TURN 107 INSERT FOR TU", "TRU17369 PINZAS DE PUNTA AGUJA 5\" MANGO", "PCD REAMER SP2003157 500.417.05849-0000", "DRILL TM400.2-NM-757259", "SP2003139 PCD COMBINATION REAMER", "5MQN11NX-054926 BORING BAR", "393.CGS-20 16 52 CYLINDRICAL SLEEVE", "393.14-20 D080X063 ER COLLET FOR TAP SHA", "930-HA05-20-090", "393.CGS-12 04 40 CYLINDRICAL SLEEVE", "393.CGS-12 06 40 CYLINDRICAL SLEEVE", "393.CGS-12 10 40 CYLINDRICAL SLEEVE", "5513 020-09 ASSEMBLY ITEM", "392.41005C-5022060 HSK TO ARBOR ADAPTOR", "930-HA05-S-12-085", "HEWC2P24AN INKCART HP 935XL HY CN", "HEWC2P25AN INKCART HP 935XL HY MG", "HEWC2P26AN INKCART HP 935XL HY YL", "299H270176 BLOCK", "HBLT90-0.98 FLAT BELTS", "51109 THRUST BALL BEARINGS", "AP-197-1-1,IVORY EMBEDDED PULLS", "C-1249-4 STAINRESS HASPS", "HOLDER BLOCK 299H544350", "GUIDE 299H544347", "LOCATING BLOCK 299H544339", "LOCATING BLOCK 2 299H262216A", "LOCATING BLOCK4 299H262218A", "PROBE BLOCK 299H030432", "COMPACTS BLOCK 299H262219A", "STOPPER 299H545322", "HOLDER 299H261215", "COMPACTS 299H254229", "LOCATING BLOCK 299H546424A", "LOCATING BLOCK1 299H262215A", "PRESS GUIDE 299H546528", "PALLETS 299H545724", "LOCATING BLOCK 299H546425", "PULLEY 299H545737", "LOCATING BLOCK 299H546124A", "LAYERING 299H546439", "UPPER PUSHER PAD 299H545231", "LOCATING BLOCK 299H546123", "LOCATING BLOCK 299H546125A", "LOCATING BLOCK 299H546122", "JIG 299H545321A", "BRACE 1 299H545821A", "BRANCE 2 299H545823", "JIG 2 299H545333", "JIG 1 299H545332", "JIG 299H544338", "STOP 1 299H545334A", "299H546530A WORK PLATE", "299H544517 WORK PLATE", "299H546421A LABEL JIG", "299H545431A JIG", "299H545723A CARRIAGE", "299H546437 ADSORB JIG", "TURBOCAST 9740 DMZ-28", "TURBOCAST 9055 DMZ-27", "FOOT 299H545630", "ARM PLATE 299H545631", "LIMIT PLATE 299H545822A", "LOCATING BLOCK 2 299H546323", "LOCATING BLOCK 3 299H546324", "BLOCK 299H546397A", "LOCATING BLOCK 299H546441", "LOCATING BLOCK 2 299H54340", "189-793 CAPACITOR RS", "JOINT SHAFT 299H261123A", "299H544224 STOP 2", "Y92A-48B TIMER COVER", "CDM2FZ20-200AZ-M9BL CILINDRO", "779113-01  NI PXI-6221 PARA USARSE COMO", "MXQ12A-307B-M9B1 MESA DESLIZANTE 12X30MM", "GDG-11107 APA 3036-39-A CORE CENTERING", "GDG-12417 CORE CENTERING APA 3009-#Ø28,0", "GDG-12416 CORE CENTERING APA 3009-A Ø55,", "GDG-12415 CORE CENTERING APA 3009-A Ø55,", "ME-12439 2544 SPRING", "299H477346 RING PIN", "490-0011 HEAT SINK RS", "299H546326 SUPPORT BASE", "299H546322A LOCATING BLOCK 1", "299H544923A CHUCK", "299H545861 BLOCK", "299H546325 LOCATING BLOCK 4", "299H545624 BRACE 1", "299H262217A LOCATING BLOCK 3", "299H544346A JIG", "299H546422 LOCITING BLOCK", "299H544342 LOCATING BLOCK 4", "299H509939 PUSH HEAD", "GDG-12409 APA 3009-B KERAMIK CORE", "4B159026 P0101-1 STRIP SHAFT PULLEY", "299H477511 PIN PARA MANDRIL", "299H477512 RING ELECTRODE", "XOMD03014-9028_GZ HOLDER-2", "XOMD03014-9011_GZ STOPPER", "RSDQA32-20DDZ-M9BL STOPPER 32 X 20 MM", "MANGUERA # PARTE - 1621 9392 00", "MANGUERA # PARTE - 1621 9550 00", "FILTRO AIRE VSD # PARTE - 1630 7783 99", "A19007M-212 WORK HOLDER (SPECIAL) AOBAGI", "DRE932 PUNTA OXIDO ALUMINIO 3/8\" PARA", "GUSANO #7099009A REAR ROTO-FLO SCR", "GUSANO TRAN.#7099010A FRONT ROTOFLOW", "CABEZAL Z4M PLUS G79057M ZEBRA", "MOLD SHIELD DRY RUST PREVENTIVE 42910A", "CILINDRO CG1GN20TN-19-XA13-CDN297", "GRIPPER CAD09-039_01/02", "#1901PRECISION  HOBBY KNIFE,LIGHHI DUTY", "#1920 HOBBY KNIFE BLADES 5BLADES/PK", "RING JIG 299H477511", "DIAMOND V-BLOCK 8MM MICAFIL # 329311", "PROTECTOR TERMICO #26659107 , XTOB2P4BC1", "I  P R)CAVITY SIDE PIN DETALLE#29", "SILDE DETALLE#32 END KEIPER 24049412-13", "INSTRUCTIVOS #52420891", "SENSOR TIPO REED #D-M9BL", "FUSIBLE 690 V. 25 A #V420000053", "FUSIBLE 250 V. 400 MA. #V42000039", "40 CHECK RING #JA435796A4", "23955842 PLUG 2721 (4P-30A)AC250V>", "THERMOCOPLE PARA NARIZ #JA755179A4", "RESISTENCIA #JA778046A4 1950W 250V", "BALERO 24MM,DIA INT, 9MM ANCH.SKF 609 2Z", "ANVIL 1/2\" AMETCH Y5A90002", "TORNILLO HEXAGONAL GRADO 8 16X2.00X90 MM", "ELECTRO VALVULA MCA ARO24 V # S5SS9D-1-G", "EXPULSOR #29  #471.016-403", "CUSTOM TORPEDO CTP-20158949", "BP40A.500BACK PLATE 40 9.5 RUNR.500", "40 SEAL RING # JA430390A4", "TIP, 1/2\"UNIVERSAL UNDERCUT  Y5A90029", "SONOTRODO # HU71.049/1 DWG 100.101.368", "CYLINDRICAL FIXTURING MAGNETOS #81745879", "HORN 1/2\" AMTECH BRANSON Y4A90023", "TARJETA,COMPACTLOGIX16   1769IQ16", "AGUJAS:  304 SS. 19 GAUGE, .032\"ID,.042\"", "EXPULSADOR # 9  471.015-316", "EXPULSADOR # 13  471.015-319", "TIP 20GA PPS .09X.5 PINK #7018205", "PROSESS FILTER #29901719", "MARCADOR PHANO AMARILO -DTM2079", "CEPILLO NO CONDUCTIVO MU HICOMP 87P0329", "PAPEL BOND T/C H1-PRO DE 75 GR 92%BLANCO", "CINTA 6200 HIGHLAND 19X33X3/4\" 3ME6200-1", "HEATER NOZZLE #26000739", "TOLOMATIC SWITCH # 8100-9089", "SOBRE BROCHE 9X12 CAFE 32# 1UNV41907", "GRAPA STD C/5000 UNV79000", "NOZZLE TIP NYL  #101479", "CABEZAL IMPRESORA ZEBRA # G79800M", "RIBON ZEBRA 5095BK04045", "MANDIL DE MEZCLILLA C/CARNAZA 60X90", "NEW PCD TIPPED V-BLOCK #G62941", "NEW PCD TIPPED V-BLOCK #G62931", "NEW PCD TIPPED V-BLOCK #G62942", "CATRIDGE CHISEL 4,8X1,5 HTS1  C245908", "CATRIDGE CHISEL 1,8X0,8 C245944(PUNTAS)", "CERAMIC PULLEY (OLD ID M912018)MSC-CP-M", "ONE WAY ROLLER BEARING #2489K12", "RESORTE COMP. RC- .719-.075-2-342 LE.190", "RESORTE RC.-.187-.021-.919 PEE LE .048", "CARBON BRUSH 0.394\"X0.630\"X1.250", "FILTRO:COLOTH,S3 FEEDMAX,FF-622#F101-329", "NON-TORQUE MSC-N912019", "PUNTA PHILLIPS P1 3-1/2 APEX 491-B (AUTO", "BALERO RADIAL 697-2Z", "PUNTA PH1 APEX 491X HEX BIT PHILLIPS 1X", "ROLLO DE SOLDADURA P/D.L#(24-9574-1404)", "CILINDRO ADVU-25-10-A-PA1 156609", "ALMOHADILLA CON ALCOHOL #54845T29", "SENSOR SMC D-M9NL", "RESORTE RC-.764-.075-3.679 PEE LE .190", "RESORTE RC .600-.070-.900 PEE LE .100", "FLEXIBLE SHAFT 1/2\"X1/2\"X 1 3/4\"#6259K31", "ACEITE 3-1 90ML DM-823", "PISTON SLT-6-10-P-A 170549 EDO2", "ALUMINUM HELUCAL FLEXIBLE #6208K569", "FIBRA OPTICA FU-49U", "SENSOR #QS18VP6LAFQ 75910", "MOTOR BALDOR BSM90A-1150AA #00537004", "SENSOR #BMF005K     30SK-C-2-SA-549-00,2", "SENSOR MAGNETICO SMC (D-M9PL)", "TUGNSTENO .315 X .394 X 12  S100W", "CNZ COSTUM NOZZLE SERIAL 51786119-10", "UNION REDUCCION DE 1/4-5/16 #Q2H07-09A", "NEOMATICS ELECTROVALVULA MODELO 226-749", "PISTON PARA CONVEYOR #1815-0934", "VALVE PIN CYVPTY042000 TOOL #2012070919", "BASE P/RELEVADOR MINIAT.D/(5VDC) 2980238", "CERAMICA BACK SIDE L1 (119710)", "CERAMICA FRONT SIDE L1 ( 119711 )", "FIXTURA PARA NIDO 4998.05-D022", "FIXTURA PARA NIDO 4998-005-D013", "MB1J2AN3-B12 WATLOW  1.5\"X2.0\" 200V/900W", "PUNTAS APLICADORAS #98385 14GA WHT TIP", "KIMTCH PURE CRITICAL TAK WIPES#06179 CL5", "MASCARILLA P/SOLDADURA (MOLDEX 2310 N99)", "CERAMICA BACK SIDE L2 (119898", "CERAMICA FRONT SIDE L2 (119899)", "MARCADOR ROJO UNI PAINT PX-20 (2997)", "CHUCK CLAW 1 4B184039P0101-0", "SPRING 4B13097500P01-0", "BEARING ROLLER GUIDE YUASA #A609020", "TEMPORARY STOND 3B309491P0101", "DIGI FORCE #9310-V001", "PUNTAS PROBE TECLOCK ZS-909", "PUNTAS PROBE TECLOCK ZS-908", "BOSCH LINER #R044229301", "SENSOR  SMAT-E8-S50-IU-M8 #540191", "TARJETA NI PCI-6221,37-PIN (779418-01)", "CILINDRO 32X30MM CDQ2B32-30DZ-XC9", "DISCO ABROSIVOS  FALCON WG90 RBC.035", "COLLECTION BAG 70195T65", "ASS JOBBER (BROCA) 2.25MM MT56-13039", "MORSE SOLID CARBIDE END MILL MT32-90822", "SOLID CARBIDE SE,CC 1-1/2 MT32-90702", "HSS JOBBER MET. 1.75MM MORSE MT56-13029", "BROCA 6.40 MM BLACK OXIDE MT56-13091", "BROCA BLACK OXIDE MT56-13139 12.50 MM", "FYLER  DAW-10191", "LBC LOADCELL #LBC-2K(321059)2000 LB", "SOLID CARBID SE ,CC,2-2/14OAL MT32-90820", "BROCA BLACK OXIDE MT56-13126 9.30 MM", "TOOL BALANCIN GR62410005 (6HH09) BD-05", "ETIQUETA ROJA FORMA F831.09X C/ ADHESIVO", "COUPLING MIKI PULLEY SGC-0405A2-6B-19B", "COUPLING NBK XGT-44C-14*19", "SWITCH NEUMATICO (SC06-1293) PNEUMADYNE", "SENSOR ACCESORY #E39-563", "ELECTRODOS  1  #211J116291", "PEGAMENTO FIXOL 40ML (DM-795)", "BROCA DE CARBURO 5/32 #AQT-30398", "RESORTE #RC 246-022-720 PE LE 094", "RESORTE #RC 240-022-1250 PEE LE 0.90", "BRUSH TIP HIGH FLOW STIFF (7018495)", "RETAINER BODY 320Z (7013900)", "CARTUCHO DE TONER NEGRO (HP-Q5949A)", "SEALING HEAD & SCREW: 725D #7020935", "DIAPHRAGM: 725D & 725DA #7020925", "2K KIT 4X0 REPAIR TTT (7704096)", "2K KIT 4X0 REPAIR TPV (7704095)", "REALAY PANASONIC DC24V 2 POLE AHJ922206", "ELECTRODE 2   211J116292", "RESORTE #RT.767-072-3.200 PEE LE.195", "CINTA DE TELA GRIS 2\" 950", "APPLIED MOTION STWPPER MOTOR  HT23-397", "PIEDRA PARA PULIR #020490", "COLLET  #L93095-C5776", "LIFT CHUCK  #F84315-C5779", "LIFT CHUCK  #K88905-C5776", "ELECTOR PIN METRIC 9/64X10\" #EP14L10", "ELECTOR PIN  2\" 3/32 X10\" #EP09L10", "ELECTOR PIN  2\" 3/32 X 6\" #EP09L06", "ELECTOR PIN  3/32 X 10\" #EP09L10P", "LOCTITE 983194 PENOMATIC CRTG.KIT", "VALVE LOCTITE 079340-1147763", "POGO PIN # CP35-E90-SPL", "POGO PIN  #LS504R-409-G-7.0", "CAMISA PARA POGO PIN #LS093RCD-01", "CARTUCHO 3/4 P/ETIQUETADORA #M21-750-499", "TRANSDUCSER TYP,TLH 225 ARD.NR. 025309", "BELT, STERLING #A6Z16-074012 #211-931", "CONECTOR DB9 HEMBRA #500-109", "CONECTOR DB9 MACHO #500-009", "CONECTOR DB9 HMBRA #500-115", "CUBIERTA PLASTICA DB9 #500-409", "V-BLADE-R=0.50-P/N 0033958", "EMPUJADOR MECANICO 203H143229", "TAPONES MECANICOS 203H143259", "FIXTURA BACE PARA MOTOR 299H121315A", "FIXTURA DE GOLPETEO   299H12130", "BLOCK MECANICO   299H128117", "PORTA PINS DE PRUEBA 228H018319B", "TUBE 1/4IN X 33 FEET B 97972", "FIXTURA PARA COLOCAR MOTOR 299H128118A", "RELEVADOR 24VDC/FONDER 55.34.9.024.5040", "BASES PARA RELEVADOR 24VDC 94140SMA", "PISTON BIMBA BORE X8.00 STROKE 32907", "OLED DISPLAY MODULE #T5950001", "CLAMP FORCE SENSOR#70962142 (SA215207A3)", "SOCKET ODAWARA DAW 43499", "BALERO PARA FLYER ODAWARA 4979", "RECVD SPACER COLLAR FLYER DAW - 43239", "POLLEY HSG COVER, CUBIERTA DAW-45199", "NIDO DE ENGRANE  20IH095248B", "DISCO DE DIAMANTE 7X1/2X11/4\" #215973", "PORTA RING DE DELRING 20IH095219A", "FIXTURA PARA PINS  #299H121221A", "PORTA PINS DE DELRING 20IH095220B", "FIXTURA PORTA PINS  #299H1213204", "PORTA PINS  299H121324A", "RELEVADOR DE SEGURIDAD #BE5982-02", "RESORTE  RC 390-042-01.225 PE LE .105", "BALERO THK HSR20A1SS  CSN:20112012200900", "RADIAL SPRAY VALVE #7021649", "V-BLADE R=0.00 UPPER #0030297", "V-BALDE R=0.00 UPPER #0037943", "BRASS BRUSH #100942", "TOUCH BUTTON OTBVP6 #28589", "SENSOR LASER Q3XTBLD-Q8 (91638)", "MODULO BANER #IM-T-9A  (61425)", "VELCRO NEGRO 1VEK90083", "TARJETA NI USB-6008    77905.01", "TARJETA NI     USB-6525   779640-01", "TARGETA NI PCI-6224   779067-01", "TARJETA NI    PCI-6221   77906601", "TARJETA NI  USB-6211   77967601", "TARJETA NI    PCI-6220   779065-01", "SENSOR   D-M9BVL", "FLIER BRG HUB RH DERECHO 202-595-01", "GRL. PURPOSE CLANER# 000-955-016 DM-804", "METAL CLEANER 1 #100-955-824 (DM-806)", "FLIER PULLEY SPACER   #DAW42899", "DEREELER DANCER PULLER #2902", "RELEVADORES  #13M4490 (60.12.9.024.0040)", "CILINDRO 40X100MM #C965DB40-100", "TORX BIT,1/4 T25 SIZE 2.75\" 7396A34", "TORX BIT,1/4 HEX T6 SIZE 2\" 7396A74", "SCVA90---00140 SHIELED FLAT CABLE", "MB0909181-4 CABLE GROUNDING,TIG,4M", "EBM PAPST 4606N AXIAL FAN (88K2739)", "DREEL WIRE CLANER CLIP #202-219", "BELT  #2915", "RELAY CR4395-EH-120-110-A-CD-ELR-I,CR", "MOTOR ASSY,LOADER S3,110V F9-240", "SCREW 10-32X1/2 #92220A173", "O-RING ID. 42.52 X 2.62 #ZU99.00566", "EXTENSION APEX 7396A34", "PUNTASDESARMADOR APEX 49-TX-20", "PUNTA P/DESARMADOR APEX 49TX10", "P/N  96F3919  RELAY IDEC RH1B-UDC24V", "CABLE ASM VDC #11987639", "BANANA BLACK (MACHO) 39F1532", "BANDA POLY-V 260J  N/P 870349", "3C COLLET 9MMRD (3543)", "CILINDRO BIMBA N/P 091-DX", "SENSOR NO IFRM 04N15A1/L 9CSADPS26BAE90", "CILINDRO BIMBA N/P 093-D", "SPRING FOR TONGE GUIDE 4B03927800P0101-0", "BNR16G08-BMS009-P013", "YT20-001-B-40-20-2009", "003991 5250-2POWER SUPPLY 24V  120VAC", "BNR16I01-AMJ006-P019-1", "NOZZLE SHUT-OFF PIN FOR MOLD # 15192", "YT20-001-B-90-30-1009A", "BEARING ROLLER STA-L(M91209-5) MSC-CP-L", "19073 HIPOT TESTER (AC-DC-IR)", "PROA10S-0-90-FU, HI-ROTOR", "MGNR09 MGN-09 RAIL ( 900 MM ) HIWIN", "SWM048-100-ET-BOS901 SINUSWECHSELRICHTER", "GRASERAS CHICAS  N/P 6009", "MAGNET HOLDER 299H477517", "BNR19H01-AMC006-P030 CAULKING BEANBG 2", "POGO PIN # 91B0530", "90B8826  FUNDA POGO PIN EVC SPR-3W-1", "2119580-1 MECHANICAL FEED ASSEMBLY", "P/N 96F3919 RELAY IDEC P/N RHIB-UDC24V", "85769 ULTRASONIC GENERATOR ULTRAPLAST", "YT20-001-B-90-30-1027", "2119806-1 INSERT, SHEAR", "REFORM OF SCISSORS 01M-938-00-74", "GLOBE PN 116912 INTERFACE BOARD", "PIN VOVER 299H264664 SUS303", "MANDRILL #150827 RING B (089.935)", "0045191 VALVE GROUP,8 CHANNEL,SY3000-8", "8842A49 CARBIDE DRILL BIT FOR  5MM SIZE", "BNR16G08-BMY009-P001-A", "Y4A50099 PIN,ECCENTRIC", "JAW CASE (TZ894-306 )", "233.943 COUPLING FOR SCREW, WITHOUT PLAY", "FLIER BRG HUB LH IZQUIERDO 202-595-02", "079340-983722    CA VALVE HEAD CHAMBER", "WIRE GUIDE PLATE MSC-4B777799 P0101-0", "299H252111A", "G62951-1 ANGLE DRIVE BRACKET", "B G62970 SWITCH BRACKET CUT SELECT", "LOCATOR BLOCK 4B617996 P0101-1", "X0MD03014-0901/01 SILVER COATING ELECTRO", "0353316 PCB ASSY,POWERBOARD,SMDE398-901", "A19007M-224 WORK HOLDER (SPECIAL)", "A19007M-210 CHUCK SMALL CLAW (SPECIAL)", "A16011M-290DATUM E PIN (SPECIAL)", "A19007M-278 GUIDE PIN (SPECIAL)", "A19007M-416 BUMPER PLATE (SPECIAL)", "A16011M-289 DATUM E PIN (SPECIAL)", "A19007M-209 CHUCK SMALL CLAW (SPECIAL)", "TS0339-F-050", "TS0339-F-051", "TS0339-D-056", "TS0339-A-051", "TS0339-A-050", "TS0339-A-020", "TS0339-B-019", "TS0339-A-021", "TS0339-F-047", "TS0339-F-038", "TS0339-B-018", "TS0339-F-048", "JEPMC-W6090-10-E CABLE FOR A0-01 MODULES", "696ZZ1 NSK MINIATURE BEARINGS", "299H548336", "299H548391", "299H548394", "299H490772A", "299H548399", "YT20-001-B-90-30-1006", "YT20-001-B-90-30-1030A", "YT20-001-C-C-30-10-1009", "BNR19H01-AMC005-P019 CAULKING PIN STATOR", "BNR19H01-BML003-P037 CAULKING PIN BH", "MGNR09 MGN-09 RAIL ( 80 MM ) HIWIN", "6904Z NSK DEEP GROOVE BALL BEARING-STAND", "ELECTRODE 299H321945A", "ELECTRODE 299H321946B", "ELECTRODE 299H321947B", "ELECTRODE 2 299H321959", "ELECTRODE 299H321958A", "PUSHER 299H321960", "PUSHER 299H321999", "GUIDE KEY 299H477516", "PUSHER 299H480740", "COVER 299H321956", "COVER 299H321939", "PUSHER 299H480739", "BNR19H01-AMC006-P023 CAULKING BEARIN 1", "YT20-001-B-100-20-0009", "YT20-001-B-90-30-1031", "YT20-001-B-90-30-1031A", "YT20-001-B-10-02-3019A", "BNR20B01-AMY004-P059 SEGMENT BACK", "RING JIG 299H477511 (A)", "RING JIG 299H477511 (B)", "5IK90GC-60 ORIENTAL MOTOR", "T-MD925A-24-G ORIENTAL MOTOR", "FL9 FILTER ORIENTAL MOTOR", "A16011M-309 CENTER GUIDE ( SPECIAL )", "079340-985404 LOCTITE 985404 ELBW FT 1/4", "MZ9G50B GEARHEAD 50 REDCTION RATIO", "C-193-1-TAK60 INDUSTRIAL LOCKS", "M91Z90G4Y INDUCTION MOTOR 90W 200V", "6920ZZ DEEP GROOVE BALL BEARINGS", "TL053900 CAMPBELL HAUSFELD (ITEM 59DH66)", "94409A121 FINE-THREAD MEDIUN-STRENGTH", "7397N125 UNIVERSAL-THREAD RUSH-TO-CONNEC", "5469K206 ANODIZED ALUMINUM RIGHT-ANGLE", "7699N125 UNIVERSAL-THREAD PUSH-TO-CONNEC", "4429K414 LOW-PRESSURE BRASS THREADED", "97-010-01 SK-1176505 SPECIAL ORDERED", "BLOCK 228H020159", "KEY 299H477850", "CLAWS BLOCK 299H477750", "SENSOR EX-19B", "PUSHER 299H477356", "97-010-01 SEN-C50-C2GS0", "299H477330 PUSHER", "BLOCK 299H477958 URETHANE", "JIG 299H477771A", "251H034945 NAIL PLATE", "INDEX PAWL MICAFIL # 329550", "6904ZZ BEARING MFG CODE: NSK", "EP-SNOOP SNOOP-8 OZ LEAK DETECTOR DM-967", "FPQA4-P5.98-L5-B5 LOCATING PIN", "602-391662-100-01 391662 WH005 16AWG", "6949K61 FLEXIBLE GROUNDING RIBBON, 5´LEN", "EX-19EB ULTRA-SLIM SIDE SENSING THRUBEAM", "4B859745 P0101-0 CLAMP CLAW", "3B859723 P101-0 START WIRE HOLLING POST", "4B812449 P0101-0 CORE SUPPORT (4)", "K07SBK089805 (1F-05UCBL(P)-2) CABLE", "DECELERATOR VRGS-9C90-19DC19", "YT20-001-B-60-02-3019A", "005319-HB-250-2-4618 HYSTERESIS BRAKE -", "91273A392 SAME-SIZE THREAD 18-8 STAINLES", "9712K424 BELLEVILLE DISC SPRING FOR 3/8\"", "G-RAP PLS PSTE EC 250G CAN (DM-976)", "PCP/CONTROLLER CABLE 7M, ANGLE 90", "00Z581 10-8109 THERMAL GRASE (DM-979)", "FC9011 GIGABIT ETHERNET PC INTERGACE", "C-B6902ZZ BALL BEARINGS", "C-B6901ZZ BALL BEARINGS", "M9MZ90G4Y 3PH MOTOR 90MM 90W 200/220/230", "PLATE 299H545625", "STOP 2 299H545335A", "STOP 1 299H544223", "SEAL PLATE 299H546126", "299H544913B CHUCK", "299H545626B BRACE 3", "299H545141 GUIDE", "299H545824 CUSHION", "299H545623A BRACE 2", "299H544723 LOCATING BLOCK", "A840407801 JIG RING MANDRIL (A-Ø84.955)", "A840407801 JIG RING MANDRIL (A-Ø84.970)", "A840407801 JIG RING MANDRIL (B-1Ø84.985)", "TF3252-20-325-03 WELDING RING B-Ø84.970", "TF3252-20-325-03 WELDING RING A-Ø84.955", "299H477511 RING JIG ( B-1 Ø84.985 )", "P/N  94F1507  BNC 20WAG #4970 POMONA", "XOMD03014-9019/01 GZ-INPLUGPLATE", "DECELERATOR VRGS-9C90-14BK14", "P/N 90F1409 RELEY TYCO PRD-11DGO-24 VDC", "#98F2365 POGOPIN OSTBY B. PYLON P4301-1F", "SOCKET #LS093RCP-1 IDI RH3SC", "POGOPIN NEWARK 91C5031 IDI SH-3-A-7-G", "RELEY 36X1970MAGNECR.750XCXM4L-120A", "POTENTIOMETER 3988447 54086756-6", "V-BLOCK #C62374-C4439  P/TORNO", "K-INDEX PAWEL#329550", "EXTRACTORES DE SOLDADURA / HNACO879", "FLIER HUB P/N  D21839", "BLADE   #TDA080P279", "O-RING ID 5X2 FPM75.5 VA75 # AU99.00418", "O-RING ID  42X1.5 #ZU99.00630", "O-RING ID.13.48X1.78 #ZU99.00564", "O-RING ID.46.X2 #ZU99.00570", "O\" RING ID 68 X 2 # ZU99. 00569", "LUBROSEAL ID.12X16.9X2.2 #ZU99.00565", "SEAL ID. 5.5X8X3.1 FOR LSR #ZU99.00488", "O\" RING ID.17X1.5 VITON #ZU99.00485", "\" V \" SUPPORT # 3BMKX31A009070", "MOTHERBOARD #09003731", "HORN (ABS MK25 515395-02-100", "HORN (ABS XT 515395-01-100", "CONECTOR ELECTRICO EPIC 10.1950", "CONECTOR ELECTRICO EPIC 10.1940", "B.HEATER TEM.3989120 4H 9713 MBH00635", "XOMD03014-9014/01 GZ-POSITIONING AXES", "880.919 FLAT MULTI-HEAD TOOL (8X43X10)", "299H241116 SENSOR BKT", "2958A123 BLACK-OXIDE HIGH-SPEED STEEL DR", "GUIDE 2  299H214242", "MP-019LC STEREO PLUG", "HEATING COIL  NV-NF7H9CLV-G05-AB", "299H544341 LOCATING BLOCK 3", "2266232-1 OCEAN_2.0_APPLICATOR-S-106F190", "TF3252-20-325-03 WELDING RING B-1Ø84.985", "9E900030000003 DRIVING MOTOR FOR MEAS", "YT18-036-430-03-00-09 ELECTRODOS"]
  in  "ToolCribPN":u16(ring) items=["100010", "100015", "100031", "100044", "100056", "100065", "100094", "100095", "100099", "100134", "100148", "100002", "100025", "100034", "100035", "100036", "100050", "100052", "100079", "100113", "100131", "100161", "100162", "100166", "100168", "100185", "100189", "100194", "100222", "100228", "100241", "100242", "100243", "100244", "100245", "100282", "100284", "100286", "100307", "100330", "100335", "100375", "100454", "100473", "100493", "100504", "100512", "100513", "100348", "100373", "100440", "100449", "100537", "100540", "100589", "100595", "100637", "100662", "100596", "100598", "100603", "100751", "100769", "100770", "100784", "100814", "100821", "100838", "100841", "100844", "100850", "100811", "100824", "100837", "100881", "100885", "100893", "100894", "100912", "100953", "100954", "100961", "100968", "100993", "100994", "101033", "101044", "101051", "101055", "101069", "101075", "101099", "100969", "101007", "101043", "101050", "101124", "101137", "101144", "101150", "101164", "101207", "101250", "101295", "101193", "101223", "101234", "101239", "101339", "101355", "101356", "101379", "101382", "101402", "101407", "101438", "101481", "101482", "101334", "101340", "101351", "101367", "101377", "101390", "101394", "101398", "101399", "101451", "101493", "101512", "101525", "101552", "101561", "101583", "101602", "101652", "101666", "101673", "101697", "101703", "101532", "101611", "101638", "101639", "101641", "101645", "101678", "101679", "101683", "101709", "101710", "101714", "101717", "101720", "101727", "101728", "101729", "101730", "101738", "101739", "101742", "101745", "101748", "101749", "101750", "101756", "101757", "101760", "101761", "101762", "101763", "101764", "101767", "101768", "101770", "101772", "101773", "101774", "101775", "101778", "101779", "101784", "101801", "101805", "101817", "101818", "101828", "101843", "101845", "101846", "101751", "101783", "101850", "101853", "101864", "101879", "101891", "101892", "101894", "101897", "101919", "101921", "101952", "101953", "101957", "101958", "101966", "101978", "101980", "102004", "102006", "101848", "101896", "101898", "102048", "102052", "102078", "102084", "102092", "102130", "102145", "102146", "102157", "102184", "102165", "102166", "102168", "102169", "102171", "102211", "102226", "102227", "102306", "102308", "102311", "102323", "102337", "102347", "102236", "102262", "102265", "102274", "102278", "102279", "102280", "102282", "102283", "102284", "102290", "102291", "102292", "102298", "102299", "102300", "102301", "102305", "102329", "102354", "102405", "102408", "102417", "102419", "102421", "102422", "102427", "102436", "102466", "102468", "102470", "102475", "102487", "102493", "102499", "102500", "102507", "102510", "102512", "102517", "102519", "102520", "102523", "102526", "102389", "102496", "102532", "102536", "102537", "102555", "102561", "102563", "102564", "102596", "102597", "102607", "102629", "102635", "102656", "102665", "102638", "102682", "102683", "102685", "102716", "102717", "102731", "102734", "102735", "102736", "102737", "102738", "102750", "102760", "102761", "102765", "102767", "102768", "102769", "102772", "102775", "102784", "102691", "102700", "102707", "102709", "102712", "102719", "102722", "102757", "102766", "102773", "102774", "102782", "102789", "102819", "102822", "102824", "102846", "102851", "102852", "102880", "102802", "102803", "102804", "102805", "102813", "102875", "102876", "102917", "102948", "102960", "102999", "103011", "103012", "103018", "103015", "103036", "103058", "103070", "103075", "103088", "103111", "103137", "103138", "103166", "103167", "103168", "103174", "103082", "103092", "103093", "103096", "103102", "103160", "103173", "103185", "103186", "103196", "103203", "103210", "103211", "103212", "103213", "103214", "103215", "103231", "103239", "103248", "103252", "103256", "103292", "103262", "103297", "103298", "103299", "103311", "103313", "103316", "103324", "103327", "103335", "103355", "103369", "103373", "103383", "103387", "103389", "103399", "103410", "103413", "103414", "103415", "103425", "103336", "103426", "103449", "103465", "103491", "103501", "103503", "103504", "103507", "103512", "103513", "103528", "103530", "103532", "103534", "103535", "103536", "103538", "103540", "103484", "103489", "103547", "103548", "103549", "103591", "103607", "103608", "103638", "103646", "103650", "103684", "103695", "103713", "103728", "103733", "103734", "103735", "103736", "103739", "103741", "103749", "103759", "103767", "103762", "103779", "103808", "103809", "103816", "103822", "103836", "103840", "103850", "103859", "103860", "103861", "103870", "103871", "103872", "103873", "103874", "103773", "103834", "103843", "103878", "103893", "103894", "103898", "103899", "103900", "103901", "103902", "103903", "103922", "103938", "103953", "103971", "103972", "103973", "103976", "103881", "103883", "103888", "103895", "103896", "103937", "103948", "104005", "104006", "104007", "104029", "104055", "104064", "104075", "104076", "104094", "104109", "104011", "104021", "104100", "104110", "104119", "104122", "104128", "104130", "104135", "104147", "104154", "104156", "104166", "104182", "104222", "104229", "104231", "104203", "104261", "104273", "104297", "104319", "104321", "104322", "104323", "104324", "104325", "104336", "104337", "104350", "104360", "104380", "104383", "104393", "104395", "104419", "104430", "104440", "104452", "104453", "104461", "104464", "104481", "104503", "104504", "104505", "104506", "104398", "104455", "104572", "104573", "104575", "104591", "104604", "104605", "104614", "104620", "104621", "104623", "104627", "104638", "104644", "104649", "104651", "104652", "104659", "104647", "104673", "104674", "104675", "104688", "104694", "104702", "104706", "104707", "104708", "104710", "104711", "104713", "104720", "104724", "104725", "104726", "104728", "104749", "104752", "104762", "104772", "104777", "104717", "104798", "104817", "104838", "104841", "104850", "104855", "104873", "104874", "104876", "104896", "104908", "104852", "104927", "104957", "104959", "104988", "104980", "104981", "105050", "105089", "105103", "105104", "105107", "105114", "105118", "105119", "105129", "105131", "105132", "105151", "105152", "105153", "105160", "105060", "105148", "105181", "105182", "105183", "105184", "105185", "105186", "105187", "105188", "105189", "105190", "105191", "105193", "105198", "105199", "105200", "105201", "105202", "105203", "105204", "105205", "105206", "105207", "105208", "105209", "105212", "105213", "105214", "105232", "105236", "105255", "105256", "105277", "105283", "105234", "105308", "105332", "105338", "105339", "105388", "105391", "105393", "105396", "105397", "105426", "105442", "105510", "105515", "105549", "105555", "105619", "105620", "105621", "105622", "105623", "105631", "105648", "105654", "105467", "105468", "105471", "105476", "105479", "105480", "105482", "105485", "105633", "105639", "105673", "105674", "105676", "105691", "105697", "105705", "105707", "105708", "105711", "105715", "105723", "105724", "105725", "105727", "105728", "105729", "105730", "105731", "105732", "105733", "105734", "105736", "105738", "105760", "105763", "105764", "105765", "105766", "105767", "105770", "105771", "105772", "105791", "105798", "105841", "105843", "105873", "105905", "105692", "105695", "105696", "105702", "105712", "105906", "105907", "105908", "105909", "105910", "105911", "105914", "106009", "106020", "106022", "106071", "106111", "106134", "106094", "106248", "106251", "106256", "106259", "106413", "106456", "106459", "106460", "106461", "106462", "106483", "106497", "106500", "106444", "106506", "106512", "106513", "106514", "106521", "106522", "106530", "106533", "106541", "106542", "106595", "106609", "106624", "106524", "106525", "106729", "106739", "106767", "106769", "106771", "106802", "106805", "106850", "106860", "106874", "106890", "106741", "106743", "106748", "106751", "106804", "106936", "106937", "106980", "106984", "106987", "107083", "107093", "107110", "107140", "107180", "107272", "107281", "107285", "107289", "107385", "107386", "107363", "107392", "107394", "107411", "107444", "107449", "107450", "107462", "107466", "107467", "107471", "107472", "107473", "107475", "107501", "107515", "107539", "107573", "107597", "107481", "107489", "107631", "107637", "107642", "107655", "107664", "107665", "107683", "107684", "107687", "107689", "107690", "107694", "107695", "107702", "107703", "107704", "107715", "107743", "107759", "107815", "107851", "107862", "107866", "107871", "107889", "107900", "107901", "107770", "107772", "107782", "107797", "107801", "107802", "107816", "107829", "107857", "107858", "107861", "107953", "107955", "107960", "107997", "108001", "108002", "108009", "108036", "108056", "108081", "108083", "108089", "108099", "108103", "108115", "108116", "108117", "108120", "108138", "108140", "108157", "108162", "108177", "108179", "108195", "108199", "108202", "108204", "108205", "108206", "108207", "108208", "108228", "108251", "108257", "108267", "108269", "108277", "108281", "108283", "108145", "108216", "108252", "108309", "108324", "108327", "108359", "108380", "108405", "108413", "108424", "108428", "108429", "108430", "108432", "108434", "108436", "108437", "108438", "108457", "108470", "108477", "108487", "108488", "108489", "108541", "108542", "108543", "108544", "108545", "108546", "108547", "108557", "108584", "108603", "108606", "108478", "108493", "108495", "108507", "108512", "108514", "108549", "108607", "108608", "108609", "108636", "108683", "108684", "108685", "108686", "108687", "108688", "108689", "108693", "108696", "108698", "108719", "108739", "108740", "108747", "108748", "108749", "108750", "108751", "108752", "108756", "108763", "108618", "108637", "108690", "108721", "108809", "108810", "108811", "108812", "108813", "108814", "108815", "108816", "108817", "108818", "108819", "108820", "108821", "108822", "108823", "108824", "108825", "108826", "108827", "108828", "108830", "108831", "108832", "108833", "108834", "108835", "108836", "108837", "108838", "108839", "108840", "108841", "108850", "108852", "108853", "108854", "108857", "108858", "108859", "108860", "108861", "108875", "108808", "108932", "108940", "108941", "108942", "108947", "108956", "108957", "108962", "108964", "108896", "108899", "108911", "109010", "109022", "109023", "109024", "109025", "109026", "109027", "109028", "109029", "109030", "109031", "109032", "109033", "109034", "109035", "109036", "109037", "109038", "109039", "109040", "109041", "109042", "109043", "109044", "109045", "109046", "109047", "109048", "109049", "109050", "109051", "109052", "109053", "109054", "109055", "109056", "109057", "109058", "109059", "109060", "109061", "109062", "109064", "109065", "109066", "109067", "109068", "109069", "109070", "109071", "109072", "109073", "109074", "109075", "109076", "109077", "109078", "109084", "109089", "109099", "109105", "109130", "109131", "109132", "109134", "109013", "109014", "109015", "109016", "109017", "109019", "109148", "109153", "109155", "109156", "109157", "109169", "109171", "109173", "109188", "109189", "109193", "109194", "109199", "109201", "109203", "109207", "109208", "109214", "109218", "109220", "109221", "109222", "109223", "109224", "109225", "109229", "109230", "109231", "109238", "109239", "109240", "109246", "109253", "109257", "109264", "109265", "109272", "109273", "109274", "109275", "109276", "109277", "109278", "109280", "109281", "109282", "109283", "109284", "109286", "109287", "109288", "109289", "109290", "109291", "109296", "109297", "109298", "109299", "109300", "109301", "109303", "109304", "109305", "109306", "109307", "109315", "109316", "109317", "109318", "109319", "109321", "109322", "109323", "109341", "109342", "109343", "109344", "109345", "109346", "109347", "109348", "109375", "109302", "109320", "109468", "109486", "109500", "109515", "109528", "109529", "109530", "109531", "109532", "109535", "109562", "109563", "109564", "109565", "109566", "109567", "109568", "109569", "109570", "109571", "109572", "109573", "109533", "109538", "109544", "109545", "109578", "109580", "109616", "109656", "109657", "109660", "109682", "109690", "112661", "112662", "116744", "116850", "116870", "116872", "117027", "117029", "109651", "110982", "117144", "117180", "117185", "117245", "117255", "117258", "117259", "117260", "117272", "117278", "117292", "117314", "117324", "117351", "117492", "117535", "117082", "117085", "117262", "117326", "117333", "117567", "117592", "117599", "117631", "117682", "117684", "117696", "117738", "117963", "117974", "117976", "118006", "117842", "117862", "118042", "118046", "118251", "118421", "118441", "118484", "118536", "118537", "118538", "118586", "118591", "118606", "118676", "118691", "118692", "118713", "118423", "118603", "119033", "119036", "119042", "119067", "119104", "119122", "119154", "119184", "119185", "119227", "119231", "119292", "119301", "119325", "119326", "119412", "119415", "119432", "119520", "119551", "119617", "119414", "119454", "119552", "119661", "119710", "119711", "119728", "119729", "119783", "119784", "119796", "119811", "119898", "119899", "119906", "119663", "119675", "119678", "119684", "119905", "119929", "119930", "120128", "120135", "120409", "120457", "120460", "120462", "120484", "120485", "120489", "120494", "120495", "120644", "120454", "120455", "120481", "120646", "120750", "120763", "120768", "120770", "120774", "120797", "120801", "120874", "120875", "120884", "120885", "120894", "120897", "120900", "120901", "120902", "120910", "120911", "120798", "120799", "120928", "120932", "120942", "120947", "120973", "120980", "120981", "120990", "120991", "120992", "120993", "121003", "121004", "121013", "121015", "121029", "121043", "120941", "120955", "121073", "121074", "121075", "121082", "121094", "121100", "121104", "121107", "121108", "121110", "121175", "121180", "121185", "121214", "121219", "121222", "121087", "121171", "121205", "121213", "121218", "121224", "121249", "121251", "121256", "121257", "121259", "121260", "121261", "121273", "121281", "121284", "121297", "121302", "121303", "121304", "121313", "121314", "121318", "121352", "121361", "121363", "121368", "121370", "121371", "121372", "121384", "121238", "121320", "121321", "121386", "121388", "121402", "121438", "121440", "121441", "104017", "107451", "115230", "121391", "121394", "121397", "121454", "100955", "115850", "101017", "101023", "101025", "101057", "100215", "101478", "101626", "101873", "101917", "104800", "102101", "100433", "107766", "109884", "105139", "107805", "100584", "109943", "102877", "105231", "102942", "109988", "103049", "104566", "110009", "110019", "105501", "105504", "101330", "106045", "108316", "110042", "101352", "120853", "105675", "103296", "121022", "101483", "103411", "108610", "101629", "107859", "108663", "121236", "103514", "101692", "103567", "106515", "106523", "108897", "103721", "103769", "109709", "109712", "109713", "109714", "109715", "109716", "109717", "109719", "109720", "109721", "109722", "109724", "109726", "109727", "109728", "109729", "109730", "109732", "109733", "109904", "109991", "109823", "109827", "109830", "109875", "109877", "109878", "109897", "109952", "109984", "109985", "109989", "110395", "110002", "110003", "110005", "110007", "110008", "110010", "110011", "110012", "110013", "110014", "110015", "110016", "110020", "110027", "110038", "110041", "110052", "110093", "110223", "110224", "110378", "110380", "110386", "110563", "110611", "110794", "110802", "110826", "110963", "110971", "110992", "110994", "110997", "110998", "111000", "110559", "110804", "110815", "110816", "110818", "110819", "110824", "110828", "110838", "110869", "110876", "110988", "111106", "111131", "111134", "111233", "111314", "111387", "111067", "111074", "111079", "111091", "111254", "111276", "111694", "111738", "111739", "111742", "111908", "111962", "112036", "112048", "112050", "112086", "111902", "111903", "111904", "111905", "112096", "112097", "112098", "112099", "112100", "112101", "112230", "112231", "112233", "112236", "112239", "112240", "112297", "109011", "111253", "113174", "113245", "113301", "113302", "113664", "114049", "115194", "115579", "115634", "115707", "115839", "115845", "115846", "115851", "115852", "115859", "115860", "115861", "115862", "115955", "116048", "116295", "116296", "116303", "116305", "116332", "109012", "111315", "106746", "111612", "102281", "107148", "112003", "112102", "103999", "112238", "104008", "107414"]
  in  "Search Button":bool
  in  "SearchString":string
  # "Tool Crib Spare Parts Search Tool"
  # "Search Result"
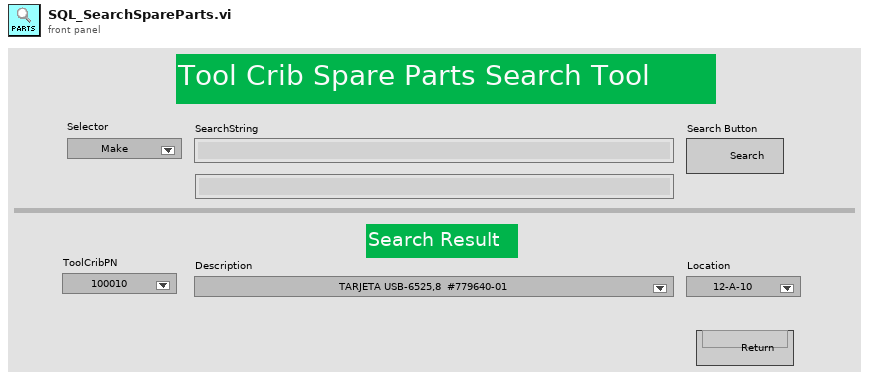
[diagram p1: front panel]
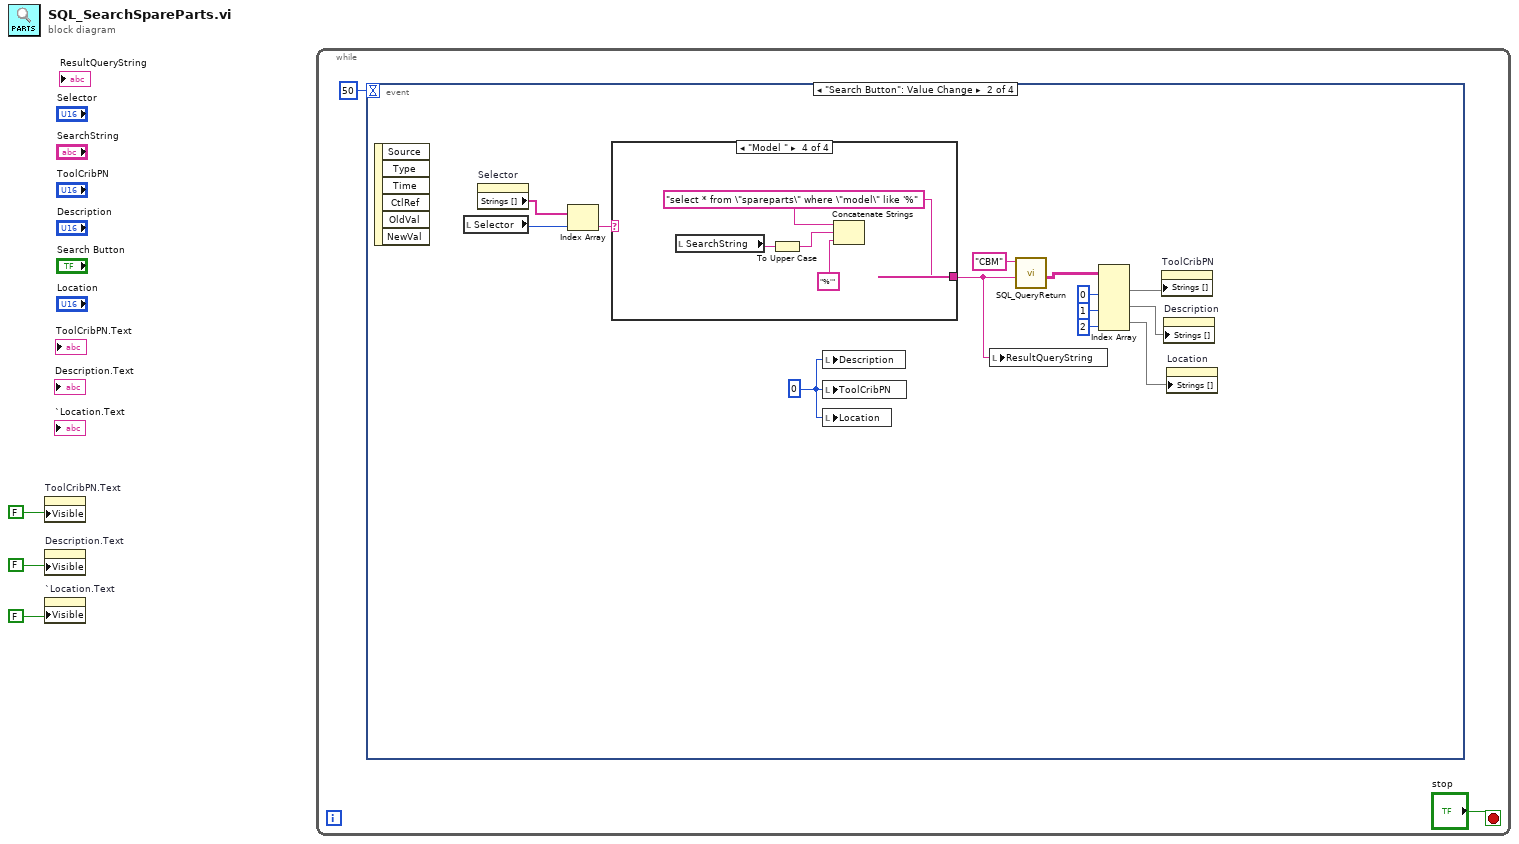
[diagram p0: block diagram]
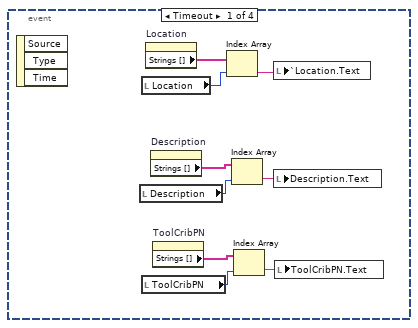
[diagram p2: hidden frame]
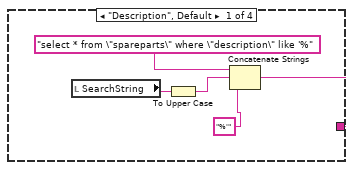
[diagram p3: hidden frame]
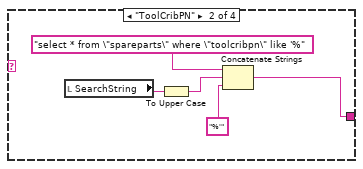
[diagram p4: hidden frame]
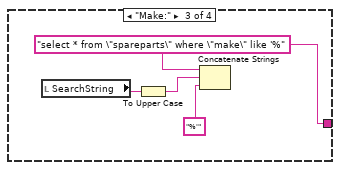
[diagram p5: hidden frame]
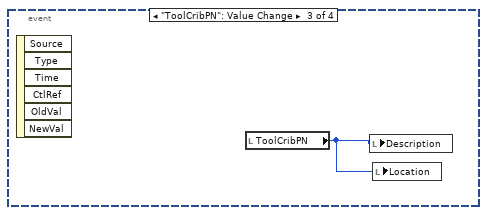
[diagram p6: hidden frame]
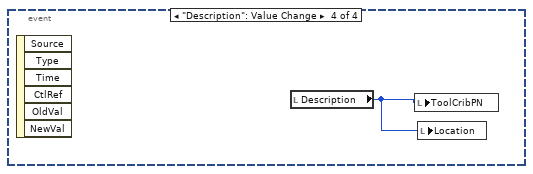
[diagram p7: hidden frame]
diagram:
  n1 = property on="ToolCribPN.Text" class="Str"("Visible"=FALSE) -> ()  [unwired: 2 in, 2 out]
  n2 = property on="Description.Text" class="Str"("Visible"=FALSE) -> ()  [unwired: 2 in, 2 out]
  n3 = property on="`Location.Text" class="Str"("Visible"=FALSE) -> ()  [unwired: 2 in, 2 out]
  n4 = while {
    stop <- "stop" stop-if-true
    n5 = event shown="[1] \"Search Button\": Value Change" {
      selector: _ -> [_ _ _ _]
      dyn-events: _ -> [_ _ _ _]
      timeout: 50 -> [_ _ _ _]
      event Timeout {
        n6 = event-data() -> ()  [unwired: 1 in, 3 out]
        n7 = local read "Description"() -> (w11:u16)
        n8 = local read "Location"() -> (w13:u16)
        n9 = local read "ToolCribPN"() -> (w6:u16)
        n10 = property on="Location" class="Ring (strict)"() -> ("Strings []"=w14:string[])  [unwired: 2 in, 2 out]
        n11 = property on="Description" class="Ring (strict)"() -> ("Strings []"=w10:string[])  [unwired: 2 in, 2 out]
        n12 = property on="ToolCribPN" class="Ring (strict)"() -> ("Strings []"=w7:string[])  [unwired: 2 in, 2 out]
        n13 = Index Array(array=w14, index=w13) -> (element=w12:string)
        n14 = Index Array(array=w10, index=w11) -> (element=w9:string)
        n15 = Index Array(array=w7, index=w6) -> (element=w8:string)
        n16 = local write "`Location.Text"(w12) -> ()
        n17 = local write "Description.Text"(w9) -> ()
        n18 = local write "ToolCribPN.Text"(w8) -> ()
      }
      event "Search Button": Value Change {
        w16 = 0
        n19 = event-data() -> ()  [unwired: 1 in, 6 out]
        n20 = local read "Selector"() -> (w27:u16)
        n21 = property on="Selector" class="Ring (strict)"() -> ("Strings []"=w26:string[])  [unwired: 2 in, 2 out]
        n22 = Index Array(array=w26, index=w27) -> (element=w25:string)
        n23 = case shown="\"Model \"" w25 {
          tunnel: [w30 w33 w38 w42] -> w15
          frame "Description", Default {
            n24 = local read "SearchString"() -> (w29:string)
            n25 = To Upper Case(1:w29) -> (0:w28:string)
            n26 = Concatenate Strings("select * from \"spareparts\" where \"description\" like '%" ("string"), w28, "%'" ("string")) -> (w30:string)
          }
          frame "ToolCribPN" {
            n27 = local read "SearchString"() -> (w37:string)
            n28 = To Upper Case(1:w37) -> (0:w36:string)
            n29 = Concatenate Strings("select * from \"spareparts\" where \"toolcribpn\" like '%" ("string"), w36, "%'" ("string")) -> (w33:string)
          }
          frame "Make:" {
            w38 = "select * from \"spareparts\" where \"make\" like '%" ("string")
            n30 = local read "SearchString"() -> (w41:string)
            n31 = To Upper Case(1:w41) -> (0:w40:string)
            n32 = Concatenate Strings(w38, w40, "%'" ("string")) -> ()  [unwired: 1 out]
          }
          frame "Model " {
            w42 = "select * from \"spareparts\" where \"model\" like '%" ("string")
            n33 = local read "SearchString"() -> (w45:string)
            n34 = To Upper Case(1:w45) -> (0:w44:string)
            n35 = Concatenate Strings(w42, w44, "%'" ("string")) -> ()  [unwired: 1 out]
          }
        }
        n36 = local write "Description"(w16) -> ()
        n37 = local write "ToolCribPN"(w16) -> ()
        n38 = local write "Location"(w16) -> ()
        n39 = local write "ResultQueryString"(w15) -> ()
        n40 = call "SQL_QueryReturn.vi"("SQL query"=w15, "ConnectionDSN"="CBM") -> ("data"=w22:string[][])  [unwired: 9 in]
        n41 = Index Array(array=w22, index (col) #1=0 ("disabled index (col)"), index (col) #2=1 ("index (col)"), index (col) #3=2 ("index (col)")) -> (element #1=w19:string[], element #2=w18:string[], element #3=w17:string[])  [unwired: 3 in]
        n42 = property on="ToolCribPN" class="Ring (strict)"("Strings []"=w19) -> ()  [unwired: 2 in, 2 out]
        n43 = property on="Description" class="Ring (strict)"("Strings []"=w18) -> ()  [unwired: 2 in, 2 out]
        n44 = property on="Location" class="Ring (strict)"("Strings []"=w17) -> ()  [unwired: 2 in, 2 out]
      }
      event "ToolCribPN": Value Change {
        n45 = event-data() -> ()  [unwired: 1 in, 6 out]
        n46 = local read "ToolCribPN"() -> (w46:u16)
        n47 = local write "Description"(w46) -> ()
        n48 = local write "Location"(w46) -> ()
      }
      event "Description": Value Change {
        n49 = event-data() -> ()  [unwired: 1 in, 6 out]
        n50 = local read "Description"() -> (w47:u16)
        n51 = local write "ToolCribPN"(w47) -> ()
        n52 = local write "Location"(w47) -> ()
      }
    }
  }
